vi "UMLEditor createWizardScriptFile.vi"(1 "localVariables":T3 {"ObjectHotspots"."HotSpot"."y" format="%.2f"; "ObjectHotspots"."HotSpot"."x" format="%.2f"; "NodesBounds"."height" format="%.2f"; "NodesBounds"."width" format="%.2f"; "NodesBounds"."y" format="%.2f"; "NodesBounds"."x" format="%.2f"; "offset"."y" format="%.2f"; "offset"."x" format="%.2f"; "gridSize" format="%.2f"; "dragStartBounds"."height" format="%.2f"; "dragStartBounds"."width" format="%.2f"; "dragStartBounds"."y" format="%.2f"; "dragStartBounds"."x" format="%.2f"; "dragStartPoint"."y" format="%.2f"; "dragStartPoint"."x" format="%.2f"; "rubberBandStart"."y" format="%.2f"; "rubberBandStart"."x" format="%.2f"; "lastMousePoint"."y" format="%.2f"; "lastMousePoint"."x" format="%.2f"; "zoom" format="%.2f"}, 2 "OnlySelectedNode(False)":bool, 5 "error in (no error)":errorcluster) -> (14 "localVariables":T3 {"ObjectHotspots"."HotSpot"."y" format="%.2f"; "ObjectHotspots"."HotSpot"."x" format="%.2f"; "NodesBounds"."height" format="%.2f"; "NodesBounds"."width" format="%.2f"; "NodesBounds"."y" format="%.2f"; "NodesBounds"."x" format="%.2f"; "offset"."y" format="%.2f"; "offset"."x" format="%.2f"; "gridSize" format="%.2f"; "dragStartBounds"."height" format="%.2f"; "dragStartBounds"."width" format="%.2f"; "dragStartBounds"."y" format="%.2f"; "dragStartBounds"."x" format="%.2f"; "dragStartPoint"."y" format="%.2f"; "dragStartPoint"."x" format="%.2f"; "rubberBandStart"."y" format="%.2f"; "rubberBandStart"."x" format="%.2f"; "lastMousePoint"."y" format="%.2f"; "lastMousePoint"."x" format="%.2f"; "zoom" format="%.2f"}, 15 "pathToScriptFile":path, 16 "Cancelled":bool, 17 "Class folder":path, 19 "error out":errorcluster)   [LabVIEW 2020]
doc: "Gets current diagram values"
uses:
  <resource>/Framework/Providers/Open_GDS/UML/UMLEditor/UMLEditor LocalVariablesType.ctl
  <resource>/Framework/Providers/Open_GDS/UML/AbstractNode_class/AbstractNode.lvclass
  <resource>/Framework/Providers/Open_GDS/UML/AbstractEdge_class/AbstractEdge.lvclass
  <resource>/Framework/Providers/Open_GDS/UML/Graphics_class/Graphics.lvclass
  <resource>/Framework/Providers/Open_GDS/UML/Grid_class/Grid.lvclass
  <resource>/Framework/Providers/Open_GDS/UML/UMLEditor/UMLEditor statesType.ctl
  <resource>/Framework/Providers/Open_GDS/UML/UMLEditor/UMLEditor tooltype.ctl
  <resource>/Framework/Providers/Open_GDS/UML/UMLEditor/UMLEditor_DiagramInfo.ctl
  <resource>/Framework/Providers/Open_GDS/UML/Graph_class/Graph.lvclass
  <resource>/Framework/Providers/Open_GDS/UML/General/Point/Point Point2D.ctl
  <resource>/Framework/Providers/Open_GDS/UML/General/Rectangle/Rectangle Rectangle2D.ctl
  <resource>/Framework/Providers/Open_GDS/UML/UMLEditor/UMLEditor ExportType.ctl
  <resource>/Framework/Providers/Open_GDS/UML/UMLEditor/UMLEditor FlattenCommandType.ctl
  <resource>/Framework/Providers/Open_GDS/UML/UMLEditor/UMLEditor ExecuteCommandType.ctl
  <resource>/Framework/Providers/Open_GDS/UML/ContextHelp/ContextHelp_EventType.ctl
  <resource>/Framework/Providers/Open_GDS/UML/UMLEditor/UMLEditor_HotSpotData.ctl
  <resource>/Framework/Providers/Open_GDS/UML/UMLEditor/UMLEditor_HotSpotType.ctl
  <resource>/Framework/Providers/Open_GDS/UML/UmlEditor_class/EventData.ctl
  <resource>/Framework/Providers/Open_GDS/UML/UMLEditor/UMLEditor GOOPWizardClassSpecification.ctl
  <resource>/Framework/Providers/Open_GDS/UML/ClassNode_class/ClassNode.lvclass
  C:/Program Files (x86)/National Instruments/LabVIEW 2020/resource/Framework/Providers/Open_GDS/UML/AbstractNode_class/AbstractNode.lvclass
  <resource>/Framework/Providers/Open_GDS/ClassProviders/Common/ScriptingFunctions/Scripting_ConnectorPanePatternType.ctl
  <resource>/Framework/Providers/Open_GDS/UML/ClassRelationshipEdge_class/ClassRelationshipEdge.lvclass
  <resource>/Framework/Providers/Open_GDS/ClassProviders/Provider_BaseClassInterface/ClassWriter_class/ClassWriter.lvclass
  <resource>/Framework/Providers/Open_GDS/UML/UMLEditor/UMLEditor_StoredPathes.ctl
  <resource>/Framework/Providers/Open_GDS/UML/InterfaceNode_class/InterfaceNode.lvclass
  <resource>/Framework/Providers/Open_GDS/UML/ContextHelp/ContextHelp_HelpTexts.ctl
  <resource>/Framework/Providers/Open_GDS/SubVIs/GOOP_ClassProviderClassType.ctl
  <resource>/Framework/Providers/Open_GDS/ClassProviders/Provider_BaseClassInterface/CreateClassData.ctl
  <resource>/Framework/Providers/Open_GDS/ClassProviders/Common/LvIcon_class/subvis/GDSLvIcon_TextDataType.ctl
  <resource>/Framework/Providers/Open_GDS/ClassProviders/Common/LvIcon_class/GDSLvIcon_WordCompressionType.ctl
  <resource>/Framework/Providers/Open_GDS/ClassProviders/Common/LvIcon_class/GDSLvIcon_TextAlignment.ctl
  <resource>/Framework/Providers/Open_GDS/ClassProviders/Common/LvIcon_class/GDSLvIcon_ClassColorTypes.ctl
  <resource>/Framework/Providers/Open_GDS/ClassProviders/Provider_BaseClassInterface/CreateInterfaceData.ctl
  <resource>/Framework/Providers/Open_GDS/ClassProviders/Provider_BaseClassInterface/ClassWriter_class/InterfaceMethodsToCreate.ctl
  <resource>/Framework/Providers/Open_GDS/ClassProviders/Common/CommonVIs/CommonVIs_AttributeType.ctl
  <resource>/Framework/Providers/Open_GDS/ClassProviders/Common/CommonVIs/CommonVIs_AttributeDataType.ctl
  <resource>/Framework/Providers/Open_GDS/ClassProviders/Common/String/GDSString_AccessScopeModifierType.ctl
  <resource>/Framework/Providers/Open_GDS/UML/ClassNode_class/ExternalSetTypes.ctl
  <resource>/Framework/Providers/Open_GDS/ClassProviders/Common/CommonVIs/CommonVIs_ClassNamePathType.ctl
  <resource>/Framework/Providers/Open_GDS/UML/ReversedEngineering/private/ReversedEngineering SyncUmlFromCodeActions.ctl
  <resource>/Framework/Providers/Open_GDS/ClassProviders/Common/ScriptingFunctions/Scripting.lvclass
  <resource>/Framework/Providers/Open_GDS/ClassProviders/Common/InterfaceLibrary/InterfaceLibrary.lvlib
  <resource>/Framework/Providers/Open_GDS/UML/UmlEditor_class/UmlEditor.lvclass
panel:
  out "Tab":enum32{"Create", "Config"}(tab)
  in  "InterfaceFolderSuffix":string="_class" caption="Interface folder suffix"
  in  "ModifyProviders":bool
  in  "Connector Pane Pattern":T1=2 items=["4x4x4", "5x6x5", "6x8x6"]
  in  "_UseLLB":bool
  in  "_CurrentClassProvider":u16(ring) caption="Class provider to use:" items=["By Reference DVR (GOOP4)", "LVClass by value", "By Reference (GOOP3)"]
  in  "Project":u16(ring) caption="Select project to add classes to" items=["Interface2.lvproj"]
  in  "Help":bool
  in  "ClassFolderSuffix":string="_class" caption="Class folder suffix"
  in  "Cancel 2":bool
  in  "CreateClasses":bool
  in  "down":bool
  in  "up":bool
  in  "ClassPath":path caption="Path for created classes (ignored for classes with a defined class path)"
  in  "Classes":T2(array[cluster])
  out "Class creation progress":i32(listbox)
  in  "Use":bool=TRUE
  out "classes":T15[](array[typedef]) {"ClassType" items=["Standard class", "Sub class from an existing base class", "Clone class from an existing class"]; "Methods"."Method Type" items=["Reading", "Modifying", "Class method - Non Modifying", "Class method - Reading", "Class method - Modifying", "Constructor", "Destructor", "Type Def"]}
  in  "ScriptfilePath":path caption="Path to store Scriptfile"
  # "LLBs"
  # "Directories"
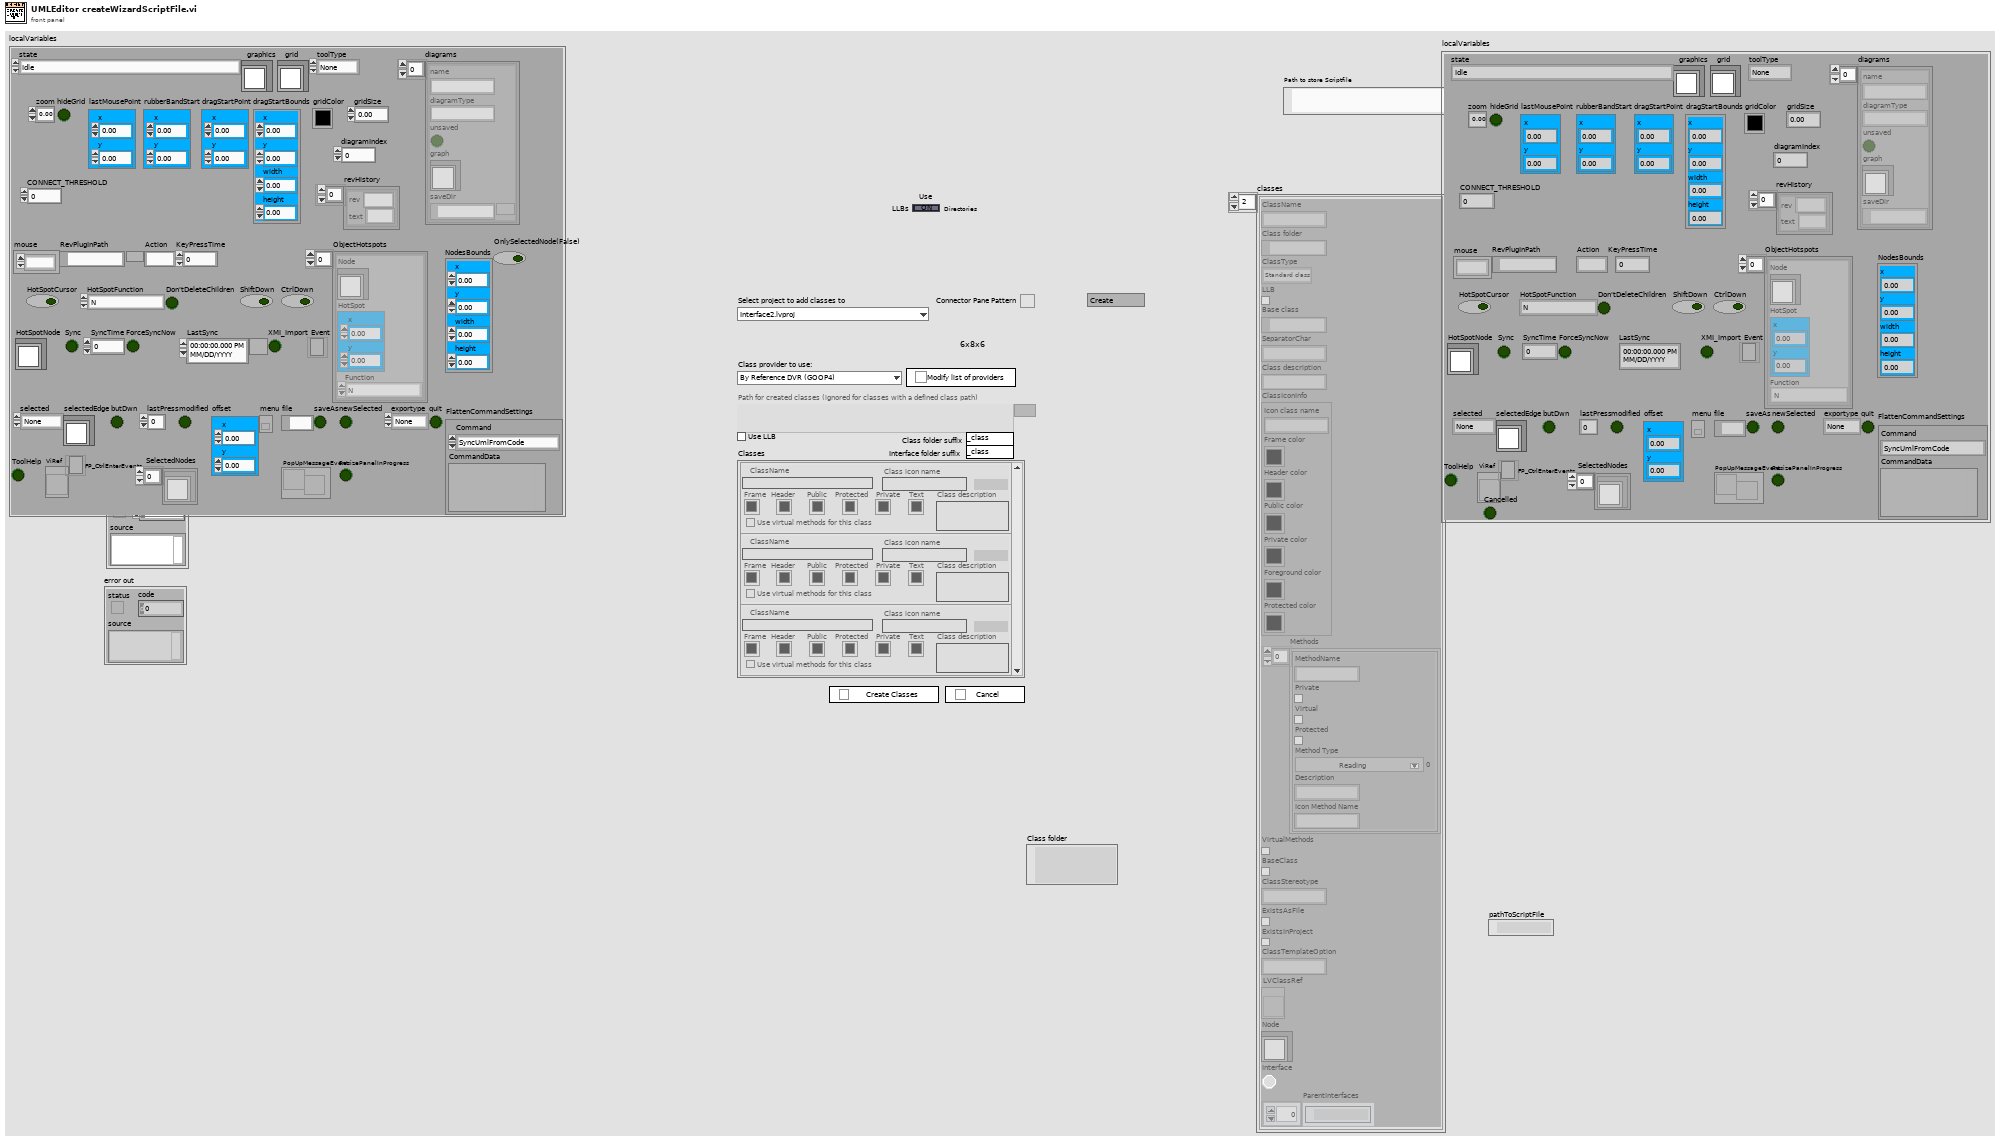
[diagram p1: front panel]
types:
  T1 = typedef "Scripting_ConnectorPanePatternType.ctl" = u16
  T2 = cluster{"ClassName":string, "Class icon name":string, "Frame":u32, "Header":u32, "Public":u32, "Protected":u32, "Private":u32, "Text":u32, "text":string, "Class description":string, "UseVirtuals":bool, "ClassIdex":i32}[]
  T3 = typedef "UMLEditor LocalVariablesType.ctl" = cluster{"state":T4, "graphics":refnum<class "Graphics.lvclass">, "grid":refnum<class "Grid.lvclass">, "toolType":T5, "diagramIndex":i32, "diagrams":T6[], "zoom":dbl, "hideGrid":bool, "lastMousePoint":T7, "rubberBandStart":T7, "dragStartPoint":T7, "dragStartBounds":T8, "gridColor":u32, "gridSize":dbl, "CONNECT_THRESHOLD":i32, "selected":T5, "selectedEdge":refnum<class "AbstractEdge.lvclass">, "butDwn":bool, "lastPress":u32, "modified":bool, "offset":T7, "menu":refnum<k9>, "file":path, "saveAs":bool, "newSelected":bool, "exportype":T9, "quit":bool, "revHistory":cluster{"rev":string, "text":string}[], "FlattenCommandSettings":T10, "PopUpMessageEvent":T12, "ResizePanelInProgress":bool, "NodesBounds":T8, "ToolHelp":bool, "ViRef":refnum<vi>, "FP_CtrlEnterEvents":refnum<event-registration>, "SelectedNodes":refnum<class "AbstractNode.lvclass">[], "mouse":refnum<k1>, "RevPlugInPath":path, "Action":string, "KeyPressTime":u32, "ObjectHotspots":T13[], "HotSpotCursor":bool, "HotSpotFunction":T14, "Don'tDeleteChildren":bool, "ShiftDown":bool, "CtrlDown":bool, "HotSpotNode":refnum<class "AbstractNode.lvclass">, "Sync":bool, "SyncTime":u32, "ForceSyncNow":bool, "LastSync":timestamp, "XMI_Import":bool, "Event":refnum<event-registration>}
  T4 = typedef "UMLEditor statesType.ctl" = enum16{"Idle", "CheckLicense", "revHistory", "Init", "Init2", "EditSelected", "RemoveSelected", "PaintComponent", "ChangeZoom", "ChangeGridSize", "Open", "Close", "Save", "ExportPicture", "Export", "Repaint", "Error", "Exit", "QUIT", "CreateScript", "ExecuteScript", "ClassReversedEngineering", "PlugInReverseEngineering", "StateReversedEngineering", "AutoPlace", "ExecuteCommand", "OpenClass", "SyncAll", "StraightenAssociation", "Copy", "Paste", "AddNodeFromProjectTree", "AddNodeFromProjectTree+SyncAll", "PanAndRepaint", "Init3", "CopyPaste", "ApplyDesignPattern", "AnalyseViInStateDiagram", "AutoSync"}
  T5 = typedef "UMLEditor tooltype.ctl" = enum16{"None", "Node", "Edge"}
  T6 = typedef "UMLEditor_DiagramInfo.ctl" = cluster{"name":string, "diagramType":string, "unsaved":bool, "graph":refnum<class "Graph.lvclass">, "saveDir":path}
  T7 = typedef "Point Point2D.ctl" = cluster{"x":dbl, "y":dbl}
  T8 = typedef "Rectangle Rectangle2D.ctl" = cluster{"x":dbl, "y":dbl, "width":dbl, "height":dbl}
  T9 = typedef "UMLEditor ExportType.ctl" = enum16{"None", "Printer", "png", "jpg", "roseUML"}
  T10 = typedef "UMLEditor FlattenCommandType.ctl" = cluster{"Command":T11, "CommandData":variant}
  T11 = typedef "UMLEditor ExecuteCommandType.ctl" = enum16{"SyncUmlFromCode", "SyncCodeFromUML", "OpenClass", "OpenFile", "CreateClass", "CreateVI", "OpenClassAttribute", "LocateInProject", "GraphExecute"}
  T12 = typedef "ContextHelp_EventType.ctl" = refnum<user-event>
  T13 = typedef "UMLEditor_HotSpotData.ctl" = cluster{"Node":refnum<class "AbstractNode.lvclass">, "HotSpot":T7, "Function":T14}
  T14 = typedef "UMLEditor_HotSpotType.ctl" = enum16{"N", "NE", "E", "SE", "S", "SW", "W", "NW", "Expand", "Collaps"}
  T15 = typedef "UMLEditor GOOPWizardClassSpecification.ctl" = cluster{"ClassName":string, "Class folder":path, "ClassType":i32, "LLB":bool, "Base class":path, "SeparatorChar":string, "Class description":string, "ClassIconInfo":cluster{"Icon class name":string, "Frame color":u32, "Header color":u32, "Public color":u32, "Private color":u32, "Foreground color":u32, "Protected color":u32}, "Methods":cluster{"MethodName":string, "Private":bool, "Virtual":bool, "Protected":bool, "Method Type":i32, "Description":string, "Icon Method Name":string}[], "VirtualMethods":bool, "BaseClass":bool, "ClassStereotype":string, "ExistsAsFile":bool, "ExistsInProject":bool, "ClassTemplateOption":string, "LVClassRef":refnum<vi>, "Node":refnum<class "ClassNode.lvclass">, "Interface":bool, "ParentInterfaces":path[]}
  T16 = cluster{"graph":refnum<class "Graph.lvclass">, "nodes":refnum<class "ClassNode.lvclass">[], "InheritEdges":refnum<class "ClassRelationshipEdge.lvclass">[], "classes":T15[], "subNodes":refnum<class "ClassNode.lvclass">[], "classGeneratorPath":path, "scriptFilePath":path, "AllNodes":refnum<class "ClassNode.lvclass">[], "CompAggEdges":refnum<class "ClassRelationshipEdge.lvclass">[], "baseNodes":refnum<class "ClassNode.lvclass">[], "Types":refnum<class "ClassNode.lvclass">[], "cancel":bool, "ClassProvider":i32, "My Computer":refnum<vi>, "ClassWriterRef":refnum<class "ClassWriter.lvclass">, "G4":bool, "Providers":string[], "InterfaceEdges":refnum<class "ClassRelationshipEdge.lvclass">[]}
  T17 = typedef "UMLEditor_StoredPathes.ctl" = enum16{"LastSearchPath", "QueuedArrayStateVI", "ClassBasePath", "ViTemplatePath", "ApplicationTemplatePath", "IniFilePath", "WizDir", "RevPlugInPath"}
  T18 = typedef "ContextHelp_HelpTexts.ctl" = enum16{"None(Hide)", "Default", "Help", "Welcome", "GettingStarted", "ClassDiagram_Help", "SequenceDiagram_Help", "UseCaseDiagram_Help", "BSelect", "BClass", "BInterface", "BPackage", "BNote", "BDependency", "BInheritance", "BInterfaceImplementation", "BAssociation", "BAggregation", "BCompAggregation", "BNoteConnector", "BObject", "BActionBar", "BCall", "BSystem", "BActor", "BUseCase", "BGeneralization", "BIncludes", "BExtends", "BUseCaseDiagramAssociation", "ClassRelationshipEdge editDialog_Bent Style", "ClassRelationshipEdge editDialog_RelationType", "ClassRelationshipEdge editDialog_Reverse association", "ClassRelationshipEdge editDialog_Start label", "ClassRelationshipEdge editDialog_Middle label", "ClassRelationshipEdge editDialog_End label", "UMLEditor reversedEngineering_Pathes", "ReversedEngineering StateReverseDialog_Help", "ReversedEngineering StateQueuedSettings_Help", "UMLEditor reversedEngineering_AddTopVIs", "UMLEditor reversedEngineering_AddClasses", "UMLEditor reversedEngineering_AddDirs", "UMLEditor reversedEngineering_Recursively", "UMLEditor reversedEngineering_Remove", "UMLEditor reversedEngineering_ClearList", "UMLEditor reversedEngineering_HideSubAss", "UMLEditor reversedEngineering_CreateTypes", "UMLEditor reversedEngineering_OnlyInheritance", "UMLEditor reversedEngineering_CreateApplication", "UMLEditor reversedEngineering_OK", "UMLEditor reversedEngineering_Cancel", "UMLEditor reversedEngineering_Help", "UMLEditor createWizardScriptFile_ScriptfilePath", "UMLEditor createWizardScriptFile_ClassPath", "UMLEditor createWizardScriptFile_Use", "UMLEditor createWizardScriptFile_PrivateDirName", "UMLEditor createWizardScriptFile_DirAppend", "UMLEditor createWizardScriptFile_Separator Character", "UMLEditor createWizardScriptFile_OK", "UMLEditor createWizardScriptFile_Cancel", "UMLEditor createWizardScriptFile_Help", "ClassNode editDialog_Class Name", "InterfaceNode editDialog_Class Name", "ClassNode editDialog_Attribute", "ClassNode editDialog_Methods", "InterfaceNode editDialog_Methods", "ClassNode editDialog_connection", "InterfaceNode editDialog_connection", "ClassNode editDialog_StereoType", "ClassNode editDialog_ShowAttrib", "ClassNode editDialog_ShowMethods", "ClassNode editDialog_ClassPath", "ClassNode editDialog_AddAttribute", "ClassNode editDialog_AddMethod", "InterfaceNode editDialog_AddMethod", "ClassNode AttributeGuide_AttributeName", "ClassNode AttributeGuide_Array?", "ClassNode AttributeGuide_Data Type", "ClassNode AttributeGuide_RefName", "ClassNode AttributeGuide_Preview", "ClassNode AttributeGuide_OK", "ClassNode AttributeGuide_Cancel", "ClassNode MethodGuide_Visibility", "ClassNode MethodGuide_Method Name", "ClassNode MethodGuide_Preview", "ClassNode MethodGuide_OK", "ClassNode MethodGuide_Cancel", "CallNode EditCallProperties_AllButtons", "ObjectNode EditObjectlProperties_AllButtons", "ActorNode EditActorProperties_AllButtons", "UseCaseRelationshipNode EditUseCaselProperties_AllButtons", "UseCaseNode EditUseCaselProperties_AllButtons", "SystemNode EditSystemProperties_AllButtons", "ReversedEngineering UpdateAttributes_AllButtons", "StateNode editDialog_AllButtons", "StateTransition editDialog_AllButtons", "ArrangeNodes Main_Picture", "ArrangeNodes Main_Zoom", "ArrangeNodes Main_Auto Zoom", "ArrangeNodes Main_shorten", "ArrangeNodes Main_Min Length", "ArrangeNodes Main_Max Length", "ArrangeNodes Main_increase", "ArrangeNodes Main_decrease", "ArrangeNodes Main_Shake", "ArrangeNodes Main", "BState", "BInitialState", "BFinalState", "BStateTransition", "StateDiagram_Help", "StateDiagram_PropertiesAllButtons", "ReversedEngineering StateReverseDialog_ClearStates", "ReversedEngineering StateReverseDialog_UseQueuedStateMachines", "ReversedEngineering StateReverseDialog_QueuedSettings", "ReversedEngineering StateReverseDialog_SearchForVIs", "ReversedEngineering StateReverseDialog_SearchCriteria", "OptionsDialog_ClassBasePath", "OptionsDialog_VIPath", "OptionsDialog_ApplicationPath", "OptionsDialog_WizDir", "OptionsDialog_IniFilePath", "OptionsDialog_DefineColors", "OptionsDialog_Help", "OptionsDialog_CreateTypes", "ClassRelationshipEdge editDialog_SplitWire"}
  T19 = typedef "GOOP_ClassProviderClassType.ctl" = enum16{"ClassWriter", "ClassReader"}
  T20 = typedef "GDSLvIcon_ClassColorTypes.ctl" = cluster{"Frame":u32, "Header Text Color":u32, "Header Background":u32, "BodyBackgroundPublic":u32, "BodyBackgroundProtected":u32, "BodyBackgroundPrivate":u32, "Body Text Color":u32, "Frame thickness":u8, "ProtectedPrivateSame":bool, "Icon Header Size":u8, "Font Compression":enum16{"Auto", "On", "Off"}, "CapitalOnly":bool}
  T21 = typedef "GDSLvIcon_TextDataType.ctl" = cluster{"Text":string, "Allow Only Capital Chars":bool, "Compression":T22, "Alignment":T23}
  T22 = typedef "GDSLvIcon_WordCompressionType.ctl" = enum16{"Auto", "On", "Off"}
  T23 = typedef "GDSLvIcon_TextAlignment.ctl" = enum16{"Center", "Left", "Right"}
  T24 = typedef "ClassWriter.lvclass/CreateClassData.ctl" = cluster{"ClassName":string, "ClassFolder":path, "ClassDescription":string, "ClassTemplateOptions":string, "BaseClass(ProjectStringPath or LvClassFilePath)":variant, "ExtraCreateParameters":variant, "FolderSuffix":string, "ParentInterfaces":path[]}
  T25 = typedef "ClassWriter.lvclass/CreateInterfaceData.ctl" = cluster{"InterfaceName":string, "InterfaceFolder":path, "InterfaceDescription":string, "FolderSuffix":string, "MethodsToCreate":T26[], "ParentInterfaces":path[]}
  T26 = typedef "ClassWriter.lvclass/InterfaceMethodsToCreate.ctl" = cluster{"Name":string, "Description":string, "MethodsArgumentsIn":T27[], "MethodsArgumentsOut":T27[], "DecendantsMustOverride":bool}
  T27 = typedef "CommonVIs_AttributeType.ctl" = cluster{"Name":string, "DataType":T28, "ArrayDim":i32, "CtrlPath":path, "DataTypeString":string, "AccessScope":T29, "InitialData":variant}
  T28 = typedef "CommonVIs_AttributeDataType.ctl" = enum16{"UINT8", "INT8", "UINT16", "INT16", "UINT32", "INT32", "UINT64", "INT64", "SGL", "DBL", "EXT", "CSG", "CDB", "CXT", "TimeStamp", "STRING", "PATH", "BOOL", "ENUM", "RefNum", "VIRefNum", "LabVIEW Class", "Cluster", "Variant", "TypeDef", "Waveform", "LabVIEW Object", "Other", "void", "Set", "Map"}
  T29 = typedef "GDSString_AccessScopeModifierType.ctl" = enum16{"public", "private", "protected", "internal"}
  T30 = typedef "ClassNode.lvclass/ExternalSetTypes.ctl" = enum16{"Name", "Attributes", "Methods", "Position", "ShowMethods", "ShowAttributes", "ClassPath"}
  T31 = typedef "CommonVIs_ClassNamePathType.ctl" = cluster{"ClassNamn":string, "ClassPath":path, "InterfaceClass":bool}
  T32 = typedef "ReversedEngineering SyncUmlFromCodeActions.ctl" = enum16{"GetAttributes&MethodsFromCode", "GetAll"}
  T33 = typedef "UMLEditor_DiagramType.ctl" = string
  T34 = typedef "BaseProvider_IniFileSettings.ctl" = cluster{"ClassFolderSuffix":string, "InterfaceFolderSuffix":string, "InterfaceIcon":string, "FileNamingOption":T35}
  T35 = typedef "BaseProvider_FileNamingOption.ctl" = enum16{"CamelCase", "Space", "Underscore"}
  T36 = typedef "CommonVIs_StereoType.ctl" = enum16{"None", "TYPE", "ENUM", "ABSTRACT", "ACTOR", "GUI", "SINGLETON", "SIGNAL", "BOUNDARY", "ENTITY", "CONTROL", "LEGACY", "APPLICATION", "VI", "LVLIB", "INTERFACE"}
  T37 = cluster{"MethodName":string, "Private":bool, "Virtual":bool, "Protected":bool, "Method Type":i32, "Description":string, "Icon Method Name":string}[]
  T38 = cluster{"MethodName":string, "Private":bool, "Virtual":bool, "Protected":bool, "Method Type":i32, "Description":string, "Icon Method Name":string}
  T39 = cluster{"ClassName":string, "Class icon name":string, "Frame":u32, "Header":u32, "Public":u32, "Protected":u32, "Private":u32, "Text":u32, "text":string, "Class description":string, "UseVirtuals":bool, "ClassIdex":i32}
  T40 = enum16{"Left Button", "Center Button", "Right Button", "Window Close"}
  T41 = enum32{"existing file", "new file", "new or existing file", "existing dir", "new dir", "new or existing dir", "existing file (use LLBs)", "new file (use LLBs)", "new or existing file (use LLBs)", "new or existing file or directory (use LLBs)"}
  T42 = typedef "ContextHelp_ShowType.ctl" = cluster{"Header":string, "Picture":picture, "Text":string}
  T43 = typedef "GOOP_WireConfigurationType.ctl" = cluster{"Edge thickness":i32, "Edge color":u32, "Center thickness":i32, "Center pattern":T44, "CenterColor1":u32, "CenterColor2":u32, "Tunnels and terminals colors":u32}
  T44 = typedef "GOOP_WirePattern.ctl" = enum16{"Solid", "Large dash", "Small dash"}
  T45 = typedef "ClassWriter.lvclass/ClassTemplateType.ctl" = cluster{"TemplateIdName":string, "TemplateUserDialogName":string, "OnlySubClassTemplate":bool, "CanDeriveFromTheseTemplateIDs":string[], "ClassSuffix":string, "Description":string, "LvLibTemplate":bool}
  T46 = cluster{"Icon class name":string, "Frame color":u32, "Header color":u32, "Public color":u32, "Private color":u32, "Foreground color":u32, "Protected color":u32}
  T47 = enum32{"invalid VI type", "Standard VI", "Control VI", "Global VI", "Polymorphic VI", "Configuration VI", "SubSystem", "Facade VI", "Method VI", "Statechart Diagram VI"}
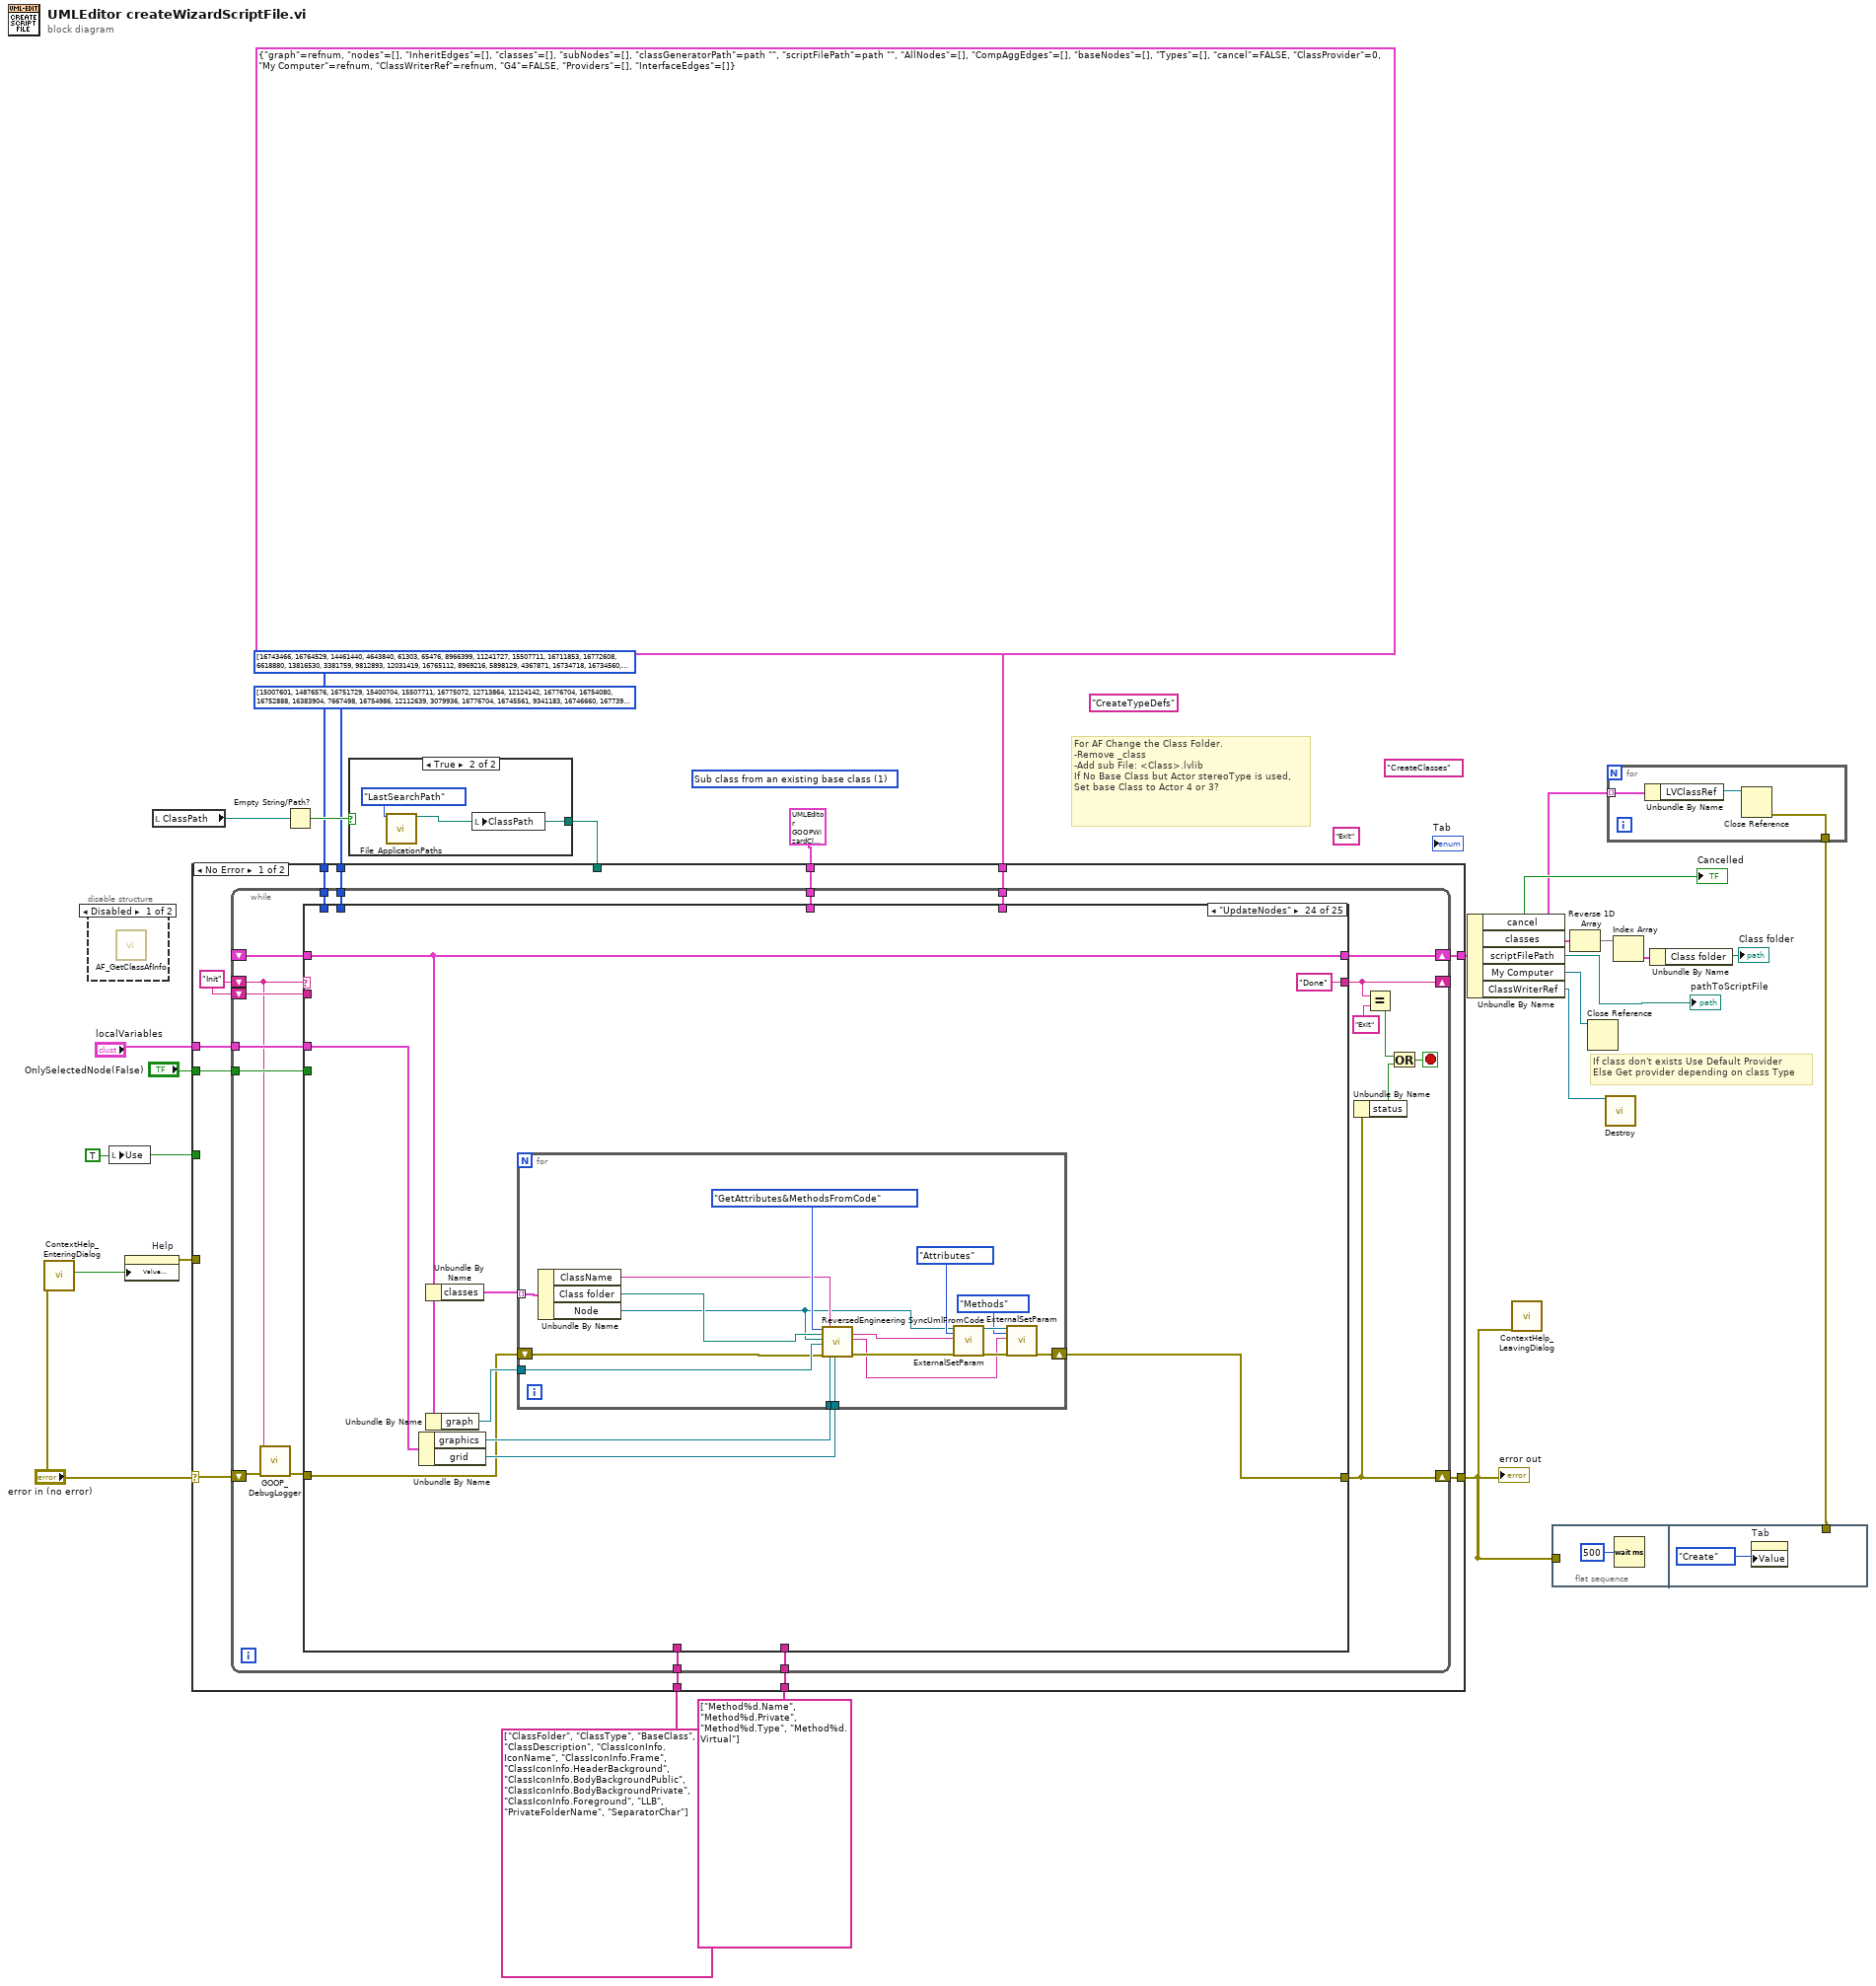
[diagram p0: block diagram]
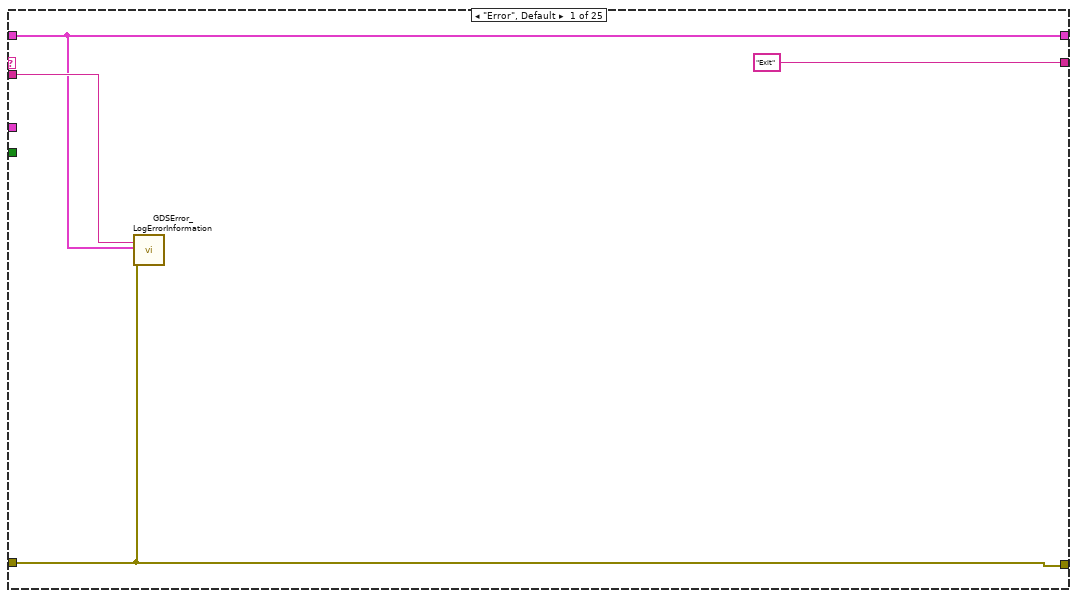
[diagram p4: hidden frame]
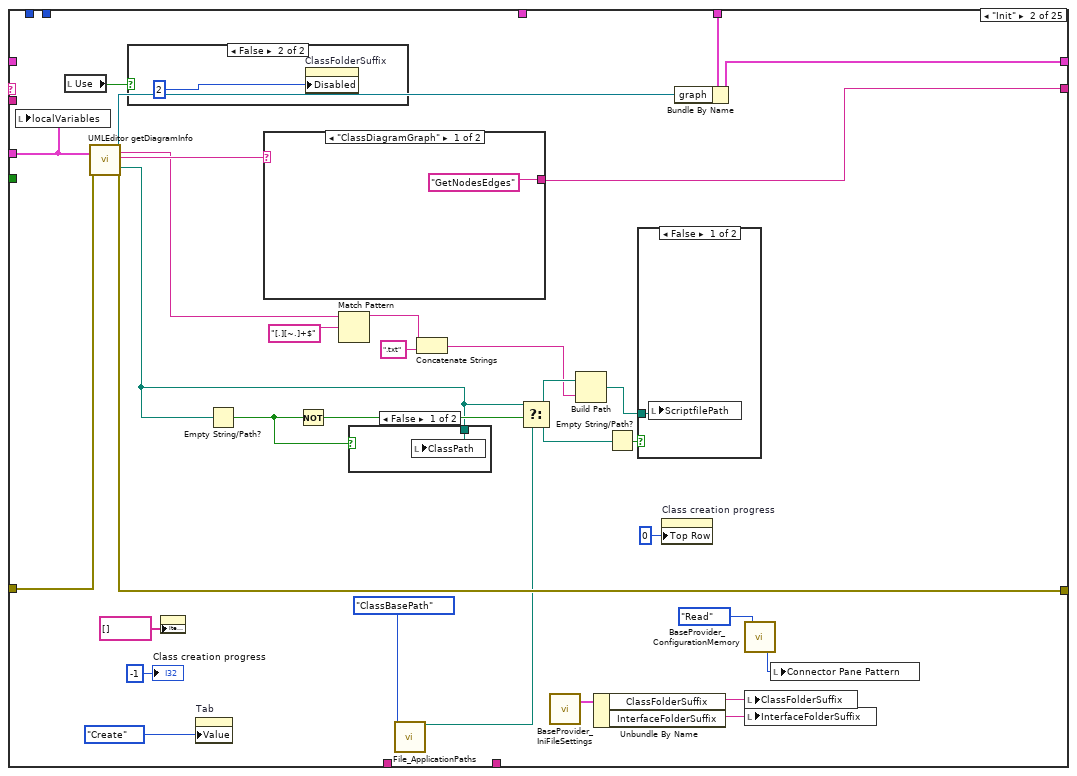
[diagram p5: hidden frame]
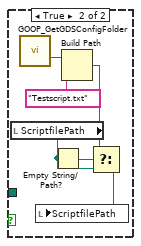
[diagram p6: hidden frame]
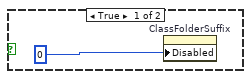
[diagram p8: hidden frame]
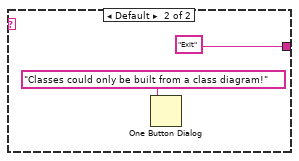
[diagram p9: hidden frame]
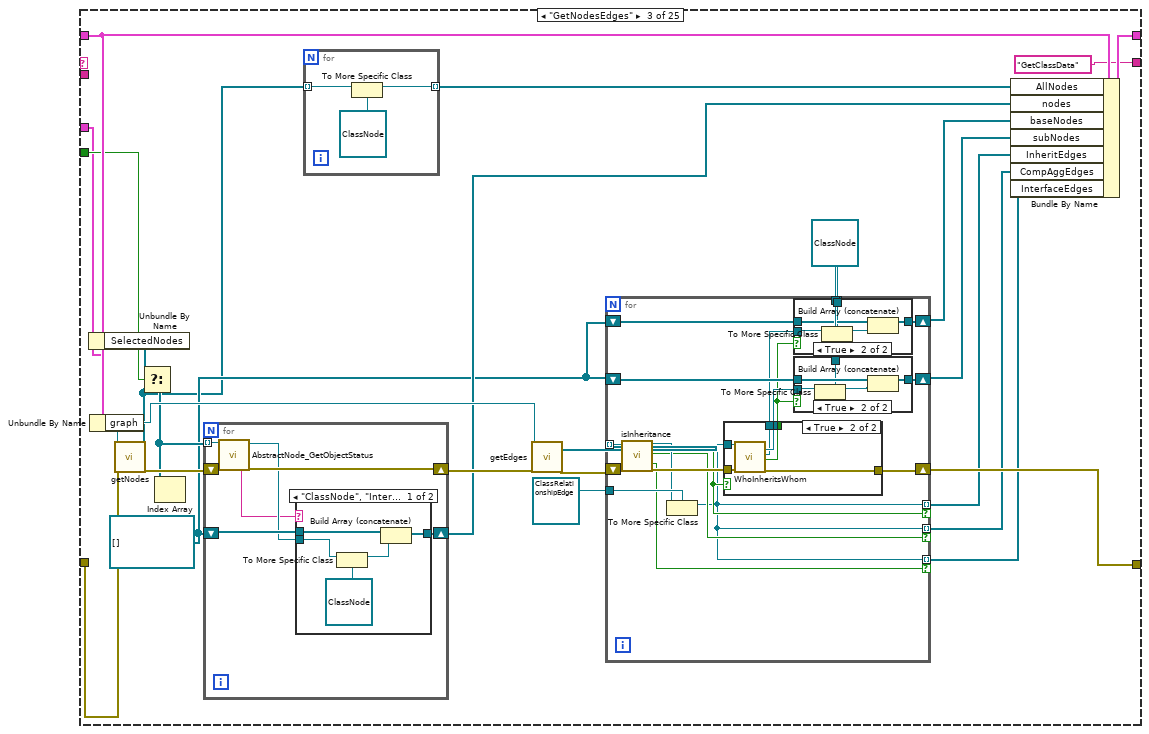
[diagram p10: hidden frame]
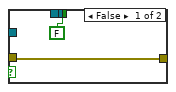
[diagram p13: hidden frame]
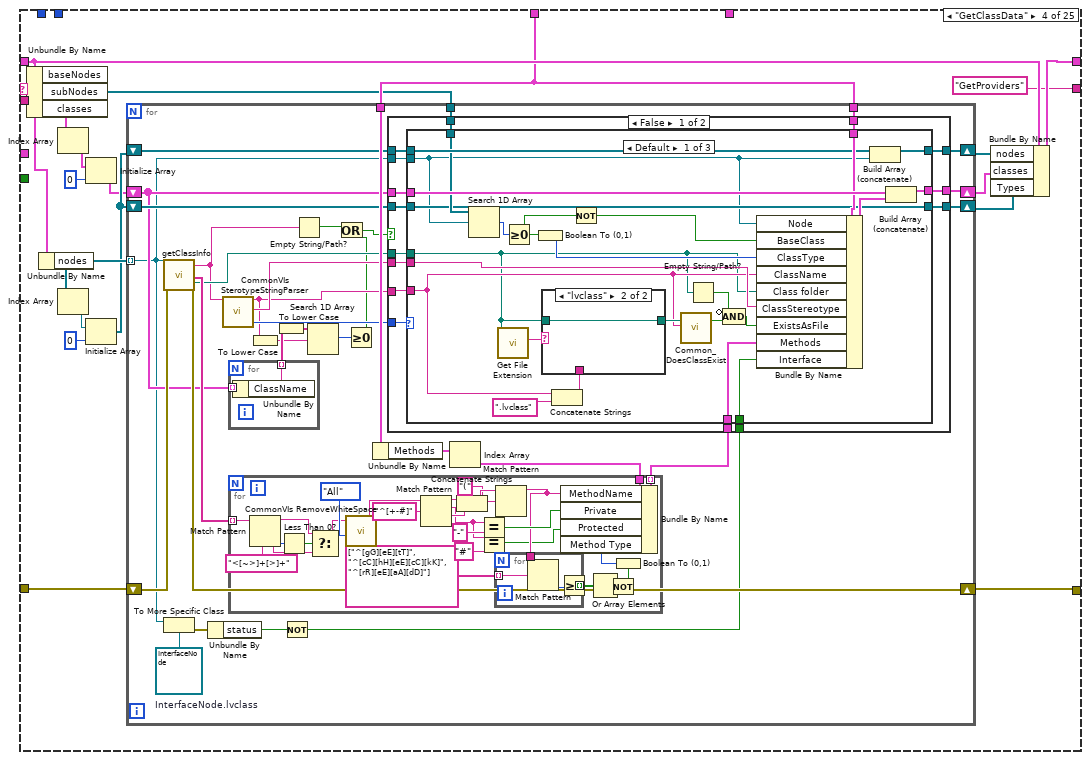
[diagram p15: hidden frame]
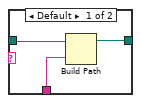
[diagram p16: hidden frame]
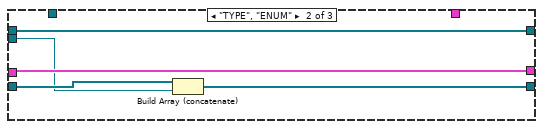
[diagram p17: hidden frame]
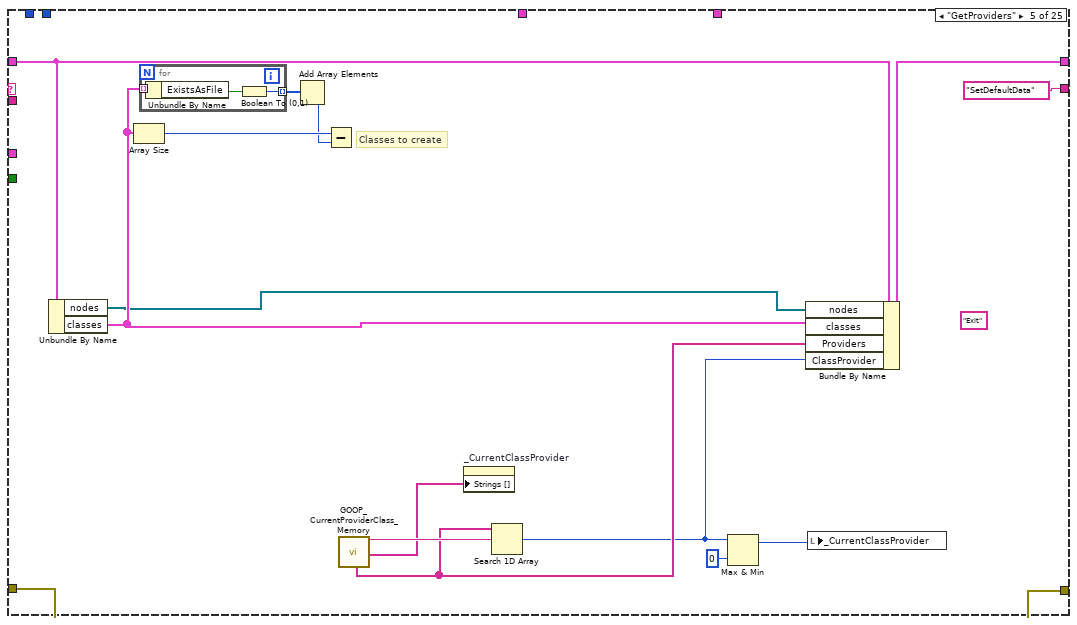
[diagram p20: hidden frame]
diagram:
  (unwired) 1 items=["Standard class", "Sub class from an existing base class", "Clone class from an existing class"] ("ClassType")
  (unwired) "CreateClasses"
  (unwired) "Exit" ("y")
  (unwired) "CreateTypeDefs" ("y")
  w8 = TRUE ("Use")
  # "For AF Change the Class Folder.\n-Remove _class\n-Add sub File: <Class>.lvlib\nIf No Base Class but Actor stereoType is used,\nSet base Class to Actor 4 or 3?"
  # "If class don't exists Use Default Provider\nElse Get provider depending on class Type"
  n1 = call <resource>:"ContextHelp_EnteringDialog.vi"("error in (no error)"="error in (no error)") -> ("HelpStatus"=w16:bool)  [unwired: 2 in, 16 out]
  n2 = disable-structure shown="Disabled" {
    frame Disabled {
      n3 = call <resource>:"AF_GetClassAfInfo.vi"() -> ()  [unwired: 6 in, 6 out]
    }
    frame Enabled {
    }
  }
  n4 = local write "Use"(w8) -> ()
  n5 = property on="Help" class="Bool (strict)"("Value (Signaling)"=w16) -> (error out=w1:errorcluster)  [unwired: 2 in, 1 out]
  n6 = local read "ClassPath"() -> (w13:path)
  n7 = Empty String/Path?(string/path=w13) -> (empty?=w12:bool)
  n8 = case shown="True" w12 {
    tunnel: [_ w27] -> w11
    frame False {
    }
    frame True {
      n9 = call <resource>:"File_ApplicationPaths.vi"("PathName"=UMLEditor_StoredPathes."LastSearchPath" ("UMLPathes")) -> ("Path Out"=w27:path)  [unwired: 3 in, 15 out]
      n10 = local write "ClassPath"(w27) -> ()
    }
  }
  n11 = case shown="No Error" "error in (no error)" {
    selector: "error in (no error)" -> [w38 w1735]
    tunnel: [w39 w1735] -> w4
    tunnel: "localVariables" -> [w40 _]
    tunnel: T15 {"ClassName"="", "Class folder"=path "", "ClassType"=0, "LLB"=FALSE, "Base class"=path "", "SeparatorChar"="", "Class description"="", "ClassIconInfo"={"Icon class name"="", "Frame color"=0, "Header color"=0, "Public color"=0, "Private color"=0, "Foreground color"=0, "Protected color"=0}, "Methods"=[], "VirtualMethods"=FALSE, "BaseClass"=FALSE, "ClassStereotype"="", "ExistsAsFile"=FALSE, "ExistsInProject"=FALSE, "ClassTemplateOption"="", "LVClassRef"=refnum, "Node"=refnum, "Interface"=FALSE, "ParentInterfaces"=[]} ("Class Info") -> [w37 _]
    tunnel: string[] ["Method%d.Name", "Method%d.Private", "Method%d.Type", "Method%d.Virtual"] -> [w36 _]
    tunnel: string[] ["ClassFolder", "ClassType", "BaseClass", "ClassDescription", "ClassIconInfo.IconName", "ClassIconInfo.Frame", "ClassIconInfo.HeaderBackground", "ClassIconInfo.BodyBackgroundPublic", "ClassIconInfo.BodyBackgroundPrivate", "ClassIconInfo.Foreground", "LLB", "PrivateFolderName", "SeparatorChar"] -> [w35 _]
    tunnel: [w34 _] -> w22
    tunnel: "OnlySelectedNode(False)" -> [w33 _]
    tunnel: w11 -> [_ _]
    tunnel: u32[] [16743466, 16764529, 14461440, 4643840, 61303, 65476, 8966399, 11241727, 15507711, 16711853, 16772608, 6618880, 13816530, 3381759, 9812893, 12031419, 16765112, 8969216, 5898129, 4367871, 16734718, 16734560, 5856767, 13140224, 16759480] -> [w32 _]
    tunnel: u32[] [15007601, 14876576, 16751729, 15400704, 15507711, 16775072, 12713864, 12124142, 16776704, 16754080, 16752888, 16383904, 7667498, 16754986, 12112639, 3079936, 16776704, 16745561, 9341183, 16746660, 16773906, 2792191, 16762993, 5766954, 16318226] -> [w31 _]
    tunnel: w8 -> [_ _]
    tunnel: T16 {"graph"=refnum, "nodes"=[], "InheritEdges"=[], "classes"=[], "subNodes"=[], "classGeneratorPath"=path "", "scriptFilePath"=path "", "AllNodes"=[], "CompAggEdges"=[], "baseNodes"=[], "Types"=[], "cancel"=FALSE, "ClassProvider"=0, "My Computer"=refnum, "ClassWriterRef"=refnum, "G4"=FALSE, "Providers"=[], "InterfaceEdges"=[]} ("local") -> [w29 _]
    tunnel: w1 -> [_ _]
    frame No Error {
      w30 = "Init"
      n12 = while {
        shift-right: [w57] -> w39
        shift-left: w38 -> [w44]
        shift-right: [w55] -> _
        shift-left: w30 -> [w42]
        tunnel: w40 -> [w60]
        shift-right: [w59] -> w34
        shift-left: _ -> [w58]
        tunnel: w37 -> [w51]
        tunnel: w36 -> [w50]
        tunnel: w35 -> [w49]
        tunnel: w33 -> [w48]
        tunnel: w32 -> [w47]
        tunnel: w31 -> [w46]
        shift-left: w30 -> [w45]
        tunnel: w29 -> [w41]
        stop <- w52 stop-if-true
        n13 = call <resource>:"GOOP_DebugLogger.vi"("error in (no error)"=w44, "State"=w42) -> ("error out"=w43:errorcluster)  [unwired: 7 in, 2 out]
        n14 = case shown="\"UpdateNodes\"" w42 {
          selector: w42 -> [_ _ _ _ _ _ _ _ _ _ _ _ _ _ _ _ _ _ w1249 _ _ w1610 _ _ _]
          tunnel: w43 -> [w61 w95 w129 w200 w336 w350 w407 w424 w470 w649 w672 w751 w913 w954 w1011 w1074 w1144 w1203 w1258 w1484 w1530 w1617 w1675 w1707 w1732]
          tunnel: [w61 w90 w128 w198 w336 w350 w407 w422 w470 w629 w672 w750 w905 w953 w1010 w1073 w1144 w1203 w1253 w1475 w1532 w1618 w1674 w1706 w1732] -> w57
          tunnel: w60 -> [_ w81 w119 _ _ _ _ _ _ _ _ _ _ _ _ _ _ _ _ w1477 _ _ _ w1705 _]
          tunnel: [w62 w92 w127 w201 w340 w361 w404 w417 w467 w644 w678 w753 w899 w956 w1012 w1075 w1142 w1201 w1252 w1472 w1538 w1615 w1677 w1708 w1733] -> w59
          tunnel: ["Exit" w93 "GetClassData" "GetProviders" "SetDefaultData" "ClassPathVisible" "CheckProject" w425 w465 "UpdatePath&Color" "UpdateBaseClasses" w742 "CheckForClassTemplateToUse(Stereotype)" ("y") "UpdateAfStereoTypeWithNoBaseClass" "UpdateAfClassTemplate" "GetParentInterfaces" "ArrangeCreationOrder" "CreateClasses" "UpdateClassPathInDiagramClasses" ("y") w1478 w1537 "FixMethods" ("y") "UpdateNodes" ("y") "Done" ("y") "Exit" ("y")] -> w55
          tunnel: w58 -> [w62 _ w126 w202 w339 w363 w405 w417 w466 w650 w677 w754 w901 w957 w1013 w1076 w1136 w1197 w1250 w1473 w1538 w1615 w1677 w1708 w1733]
          tunnel: w51 -> [_ _ _ w199 _ _ _ _ _ _ _ _ _ _ _ _ _ _ _ _ _ _ _ _ _]
          tunnel: w50 -> [_ _ _ _ _ _ _ _ _ _ _ _ _ _ _ _ _ _ _ _ _ _ _ _ _]
          tunnel: w49 -> [_ _ _ _ _ _ _ _ _ _ _ _ _ _ _ _ _ _ _ _ _ _ _ _ _]
          tunnel: w48 -> [_ _ w121 _ _ _ _ _ _ _ _ w745 _ _ _ _ _ _ _ _ _ _ _ _ _]
          tunnel: w47 -> [_ _ _ _ _ w354 _ _ _ _ _ _ _ _ _ _ _ _ _ _ _ _ _ _ _]
          tunnel: w46 -> [_ _ _ _ _ w353 _ _ _ _ _ _ _ _ _ _ _ _ _ _ _ _ _ _ _]
          tunnel: w45 -> [w63 _ _ _ _ _ _ _ _ _ _ _ _ _ _ _ _ _ _ _ w1531 _ _ _ _]
          tunnel: w41 -> [_ w70 _ _ _ _ _ _ _ _ _ _ _ _ _ _ _ _ _ _ _ _ _ _ _]
          frame "Error", Default {
            n15 = call <resource>:"GDSError_LogErrorInformation.vi"("State"=w63, "LocalVariableData"=w62, "error in (no error)"=w61) -> ()  [unwired: 1 in, 16 out]
          }
          frame "Init" {
            n16 = local write "localVariables"(w81) -> ()
            n17 = local read "Use"() -> (w84:bool)
            n18 = call <resource>:"UMLEditor getDiagramInfo.vi"("localVariables"=w81, "error in (no error)"=w95) -> ("graph"=w91:refnum<class "Graph.lvclass">, "name"=w87:string, "diagramType"=w94:T33, "saveDir"=w78:path, "error out"=w90:errorcluster)  [unwired: 13 out]
            n19 = case shown="False" w84 {
              frame True {
                n20 = property on="ClassFolderSuffix" class="Str"("Disabled"=u8 0) -> ()  [unwired: 2 in, 2 out]
              }
              frame False {
                n21 = property on="ClassFolderSuffix" class="Str"("Disabled"=u8 2) -> ()  [unwired: 2 in, 2 out]
              }
            }
            n22 = property on="Class creation progress" class="LstBox (strict)"("Item Names"=string[] []) -> ()  [unwired: 2 in, 2 out]
            n23 = property on="Tab" class="TabCtl (strict)"("Value"=enum32{"Create", "Config"}."Create" ("Tab")) -> ()  [unwired: 2 in, 2 out]
            n24 = Empty String/Path?(string/path=w78) -> (empty?=w82:bool)
            n25 = case shown="\"ClassDiagramGraph\"" w94 {
              tunnel: ["GetNodesEdges" "Exit"] -> w93
              frame "ClassDiagramGraph" {
              }
              frame Default {
                n26 = One Button Dialog(message="Classes could only be built from a class diagram!") -> ()  [unwired: 2 out]
              }
            }
            n27 = Not(x=w82) -> (.not. x?=w85:bool)
            n28 = Match Pattern(string=w87, regular expression="[.][~.]+$") -> (before substring=w88:string)  [unwired: 4 out]
            n29 = case shown="False" w82 {
              tunnel: w78 -> [w103 _]
              frame False {
                n30 = local write "ClassPath"(w103) -> ()
              }
              frame True {
              }
            }
            n31 = call <resource>:"File_ApplicationPaths.vi"("PathName"=UMLEditor_StoredPathes."ClassBasePath" ("UMLPathes")) -> ("Path Out"=w79:path)  [unwired: 3 in, 15 out]
            n32 = Concatenate Strings(w88, ".txt" ("string")) -> (w76:string)
            n33 = Select(t=w78, s=w85, f=w79) -> (s? t:f=w77:path)
            n34 = call <resource>:"BaseProvider_IniFileSettings.vi"() -> ("IniFileSettings"=w67:T34)  [unwired: 18 in, 1 out]
            n35 = Build Path(base path=w77, name or relative path=w76) -> (appended path=w75:path)
            n36 = Unbundle By Name(w67) -> ("ClassFolderSuffix"=w66:string, "InterfaceFolderSuffix"=w65:string)
            n37 = Empty String/Path?(string/path=w77) -> (empty?=w83:bool)
            n38 = case shown="False" w83 {
              tunnel: w75 -> [w96 _]
              frame False {
                n39 = local write "ScriptfilePath"(w96) -> ()
              }
              frame True {
                n40 = local read "ScriptfilePath"() -> (w98:path)
                n41 = call <resource>:"GOOP_GetGDSConfigFolder.vi"() -> ("GDSFolderPath"=w102:path)
                n42 = Empty String/Path?(string/path=w98) -> (empty?=w100:bool)
                n43 = Build Path(base path=w102, name or relative path="Testscript.txt") -> (appended path=w99:path)
                n44 = Select(t=w99, s=w100, f=w98) -> (s? t:f=w97:path)
                n45 = local write "ScriptfilePath"(w97) -> ()
              }
            }
            n46 = property on="Class creation progress" class="LstBox (strict)"("Top Row"=0) -> ()  [unwired: 2 in, 2 out]
            n47 = Bundle By Name(cluster=w70, "graph"=w91) -> (w92:T16)
            n48 = call <resource>:"BaseProvider_ConfigurationMemory.vi"("Action"=enum16{"Read", "Load", "Save", "Set"}."Read") -> ("PatternOut"=w68:T1)  [unwired: 12 in, 6 out]
            n49 = local write "ClassFolderSuffix"(w66) -> ()
            n50 = local write "InterfaceFolderSuffix"(w65) -> ()
            n51 = local write "Connector Pane Pattern"(w68) -> ()
            "Class creation progress" <- -1 ("Class creation progress")
          }
          frame "GetNodesEdges" {
            w114 = refnum<class "ClassNode.lvclass"> refnum ("reference")
            w116 = refnum<class "ClassNode.lvclass">[] [] ("nodes")
            n52 = Unbundle By Name(w119) -> ("SelectedNodes"=w122:refnum<class "AbstractNode.lvclass">[])
            n53 = Unbundle By Name(w126) -> ("graph"=w124:refnum<class "Graph.lvclass">)
            n54 = call-dynamic "getNodes.vi"("reference"=w124, "error in (no error)"=w129) -> ("nodes"=w113:refnum<class "AbstractNode.lvclass">[], "error out"=w133:errorcluster)  [unwired: 15 in, 1 out]
            n55 = Select(t=w122, s=w121, f=w113) -> (s? t:f=w123:refnum<class "AbstractNode.lvclass">[])
            n56 = Index Array(array=w123) -> ()  [unwired: 1 in, 1 out]
            n57 = for {
              shift-right: [w180] -> w132
              shift-left: w133 -> [w182]
              tunnel: w123 -> [w181] mode=indexing
              shift-right: [w177] -> w118
              shift-left: w116 -> [w179]
              n58 = call <resource>:"AbstractNode_GetObjectStatus.vi"("reference in"=w181, "error in (no error)"=w182) -> ("Class name"=w176:string, "reference out"=w178:refnum<class "AbstractNode.lvclass">, "error out"=w180:errorcluster)  [unwired: 15 out]
              n59 = case shown="\"ClassNode\", \"InterfaceNode\"" w176 {
                tunnel: w179 -> [w187 w188]
                tunnel: w178 -> [w185 _]
                tunnel: [w186 w188] -> w177
                frame "ClassNode", "InterfaceNode" {
                  n60 = To More Specific Class(target class=refnum<class "ClassNode.lvclass"> refnum ("reference"), reference=w185) -> (specific class reference=w184:refnum<class "ClassNode.lvclass">)  [unwired: 1 in, 1 out]
                  n61 = Build Array (concatenate)(w187, w184) -> (w186:refnum<class "ClassNode.lvclass">[])
                }
                frame Default {
                }
              }
            }
            n62 = for {
              tunnel: w113 -> [w135] mode=indexing
              tunnel: [w134] -> w112 mode=indexing
              n63 = To More Specific Class(target class=refnum<class "ClassNode.lvclass"> refnum ("reference"), reference=w135) -> (specific class reference=w134:refnum<class "ClassNode.lvclass">)  [unwired: 1 in, 1 out]
            }
            n64 = call-dynamic "getEdges.vi"("reference"=w124, "error in (no error)"=w132) -> ("edges"=w130:refnum<class "AbstractEdge.lvclass">[], "error out"=w131:errorcluster)  [unwired: 15 in, 1 out]
            n65 = for {
              shift-right: [w150] -> w128
              shift-left: w131 -> [w155]
              tunnel: w130 -> [w154] mode=indexing
              shift-right: [w152] -> w125
              shift-left: w116 -> [w153]
              shift-right: [w148] -> w120
              shift-left: w116 -> [w147]
              tunnel: refnum<class "ClassRelationshipEdge.lvclass"> refnum ("nodeRef") -> [w144]
              tunnel: w114 -> [w142]
              tunnel: w114 -> [w141]
              tunnel: [w138] -> w111 mode=indexing if=w140
              tunnel: [w138] -> w110 mode=indexing if=w139
              tunnel: [w138] -> w109 mode=indexing if=w137
              n66 = call-dynamic "isInheritance.vi"("reference"=w154, "error in (no error)"=w155) -> ("reference out"=w143:refnum<class "AbstractEdge.lvclass">, "isInheritance"=w140:bool, "isCompAggregation"=w139:bool, "isInterfaecImplementing"=w137:bool, "error out"=w151:errorcluster)  [unwired: 13 in]
              n67 = To More Specific Class(target class=w144, reference=w143) -> (specific class reference=w138:refnum<class "ClassRelationshipEdge.lvclass">)  [unwired: 1 in, 1 out]
              n68 = case shown="True" w140 {
                tunnel: w151 -> [w168 w175]
                tunnel: [w168 w174] -> w150
                tunnel: w138 -> [_ w173]
                tunnel: [FALSE ("inheritanceUsed") w172] -> w146
                tunnel: [_ w171] -> w149
                tunnel: [_ w170] -> w145
                frame False {
                }
                frame True {
                  n69 = call <resource>:"WhoInheritsWhom.vi"("reference"=w173, "error in (no error)"=w175) -> ("inherits"=w171:refnum<class "AbstractNode.lvclass">, "base"=w170:refnum<class "AbstractNode.lvclass">, "inheritanceUsed"=w172:bool, "error out"=w174:errorcluster)  [unwired: 14 out]
                }
              }
              n70 = case shown="True" w146 {
                tunnel: w145 -> [_ w159]
                tunnel: w147 -> [w156 w161]
                tunnel: [w156 w160] -> w148
                tunnel: w142 -> [_ w157]
                frame False {
                }
                frame True {
                  n71 = To More Specific Class(target class=w157, reference=w159) -> (specific class reference=w158:refnum<class "ClassNode.lvclass">)  [unwired: 1 in, 1 out]
                  n72 = Build Array (concatenate)(w161, w158) -> (w160:refnum<class "ClassNode.lvclass">[])
                }
              }
              n73 = case shown="True" w146 {
                tunnel: w149 -> [_ w165]
                tunnel: w153 -> [w162 w167]
                tunnel: [w162 w166] -> w152
                tunnel: w141 -> [_ w163]
                frame False {
                }
                frame True {
                  n74 = To More Specific Class(target class=w163, reference=w165) -> (specific class reference=w164:refnum<class "ClassNode.lvclass">)  [unwired: 1 in, 1 out]
                  n75 = Build Array (concatenate)(w167, w164) -> (w166:refnum<class "ClassNode.lvclass">[])
                }
              }
            }
            n76 = Bundle By Name(cluster=w126, "AllNodes"=w112, "nodes"=w118, "baseNodes"=w120, "subNodes"=w125, "InheritEdges"=w111, "CompAggEdges"=w110, "InterfaceEdges"=w109) -> (w127:T16)
          }
          frame "GetClassData" {
            n77 = Unbundle By Name(w202) -> ("subNodes"=w194:refnum<class "ClassNode.lvclass">[], "classes"=w205:T15[])  [unwired: 1 out]
            n78 = Unbundle By Name(w202) -> ("nodes"=w206:refnum<class "ClassNode.lvclass">[])
            n79 = Index Array(array=w205) -> (element=w203:T15)  [unwired: 1 in]
            n80 = Index Array(array=w206) -> (element=w197:refnum<class "ClassNode.lvclass">)  [unwired: 1 in]
            n81 = Initialize Array(w203, 0 ("dimension size")) -> (w190:T15[])
            n82 = Initialize Array(w197, 0 ("dimension size")) -> (w193:refnum<class "ClassNode.lvclass">[])
            n83 = for {
              tunnel: w206 -> [w210] mode=indexing
              shift-right: [w238] -> w191
              shift-left: w190 -> [w220]
              tunnel: w199 -> [w237]
              shift-right: [w235] -> w198
              shift-left: w200 -> [w236]
              tunnel: w199 -> [w234]
              shift-right: [w230] -> w195
              shift-left: w193 -> [w229]
              tunnel: w194 -> [w228]
              shift-right: [w224] -> w192
              shift-left: w193 -> [w225]
              w211 = refnum<class "InterfaceNode.lvclass"> refnum  # InterfaceNode.lvclass
              n84 = call-dynamic "getClassInfo.vi"("reference"=w210, "error in (no error)"=w236) -> ("className"=w223:string, "methods"=w227:string[], "ClassPath"=w226:path, "error out"=w235:errorcluster)  [unwired: 8 in, 6 out]
              n85 = To More Specific Class(target class=w211, reference=w210) -> (error out=w209:errorcluster)  [unwired: 1 in, 1 out]
              n86 = Unbundle By Name(w209) -> ("status"=w208:bool)
              n87 = call <resource>:"CommonVIs SterotypeStringParser.vi"("SterotypeStringIn"=w223) -> ("StereoType"=w221:T36, "Name"=w217:string, "Sterotype"=w222:string)  [unwired: 16 out]
              n88 = for {
                tunnel: w220 -> [w240] mode=indexing
                tunnel: [w239] -> w219 mode=indexing
                n89 = Unbundle By Name(w240) -> ("ClassName"=w239:string)
              }
              n90 = To Lower Case(string=w217) -> (all lower case string=w216:string)
              n91 = To Lower Case(string=w219) -> (all lower case string=w218:string[])
              n92 = Not(x=w208) -> (.not. x?=w207:bool)
              n93 = Empty String/Path?(string/path=w223) -> (empty?=w214:bool)
              n94 = Search 1D Array(1D array=w218, element=w216) -> (index of element=w213:i32)  [unwired: 1 out]
              n95 = Greater Or Equal To 0?(x=w213) -> (x >= 0?=w212:bool)
              n96 = Or(x=w214, y=w212) -> (x .or. y?=w215:bool)
              n97 = Unbundle By Name(w234) -> ("Methods"=w233:T37)
              n98 = Index Array(array=w233) -> (element=w232:T38)  [unwired: 1 in]
              n99 = for {
                tunnel: w227 -> [w320] mode=indexing
                tunnel: w232 -> [w319]
                tunnel: [w318] -> w231 mode=indexing
                n100 = Match Pattern(string=w320, regular expression="<[~>]+[>]+") -> (before substring=w300:string, after substring=w301:string, offset past match=w302:i32)  [unwired: 2 out]
                n101 = Less Than 0?(x=w302) -> (x < 0?=w303:bool)
                n102 = Select(t=w300, s=w303, f=w301) -> (s? t:f=w299:string)
                n103 = call <resource>:"CommonVIs RemoveWhiteSpace.vi"("Remove from"=enum16{"Begining", "End", "Beg+End", "All"}."All", "String in"=w299) -> ("String out"=w317:string)  [unwired: 2 in, 3 out]
                n104 = Match Pattern(string=w317, regular expression="^[+-#]") -> (before substring=w315:string, match substring=w298:string, after substring=w314:string)  [unwired: 2 out]
                n105 = Concatenate Strings(w315, w314) -> (w306:string)
                n106 = Equal?(x=w298, y="-") -> (x = y?=w312:bool)
                n107 = Equal?(x=w298, y="#") -> (x = y?=w296:bool)
                n108 = Match Pattern(string=w306, regular expression="(") -> (before substring=w304:string)  [unwired: 4 out]
                n109 = for {
                  tunnel: [w325] -> w311 mode=indexing
                  tunnel: w304 -> [w324]
                  tunnel: string[] ["^[gG][eE][tT]", "^[cC][hH][eE][cC][kK]", "^[rR][eE][aA][dD]"] -> [w323] mode=indexing
                  n110 = Match Pattern(string=w324, regular expression=w323) -> (offset past match=w326:i32)  [unwired: 4 out]
                  n111 = Greater Or Equal To 0?(x=w326) -> (x >= 0?=w325:bool)
                }
                n112 = Or Array Elements(Boolean array=w311) -> (logical OR=w310:bool)
                n113 = Not(x=w310) -> (.not. x?=w309:bool)
                n114 = Boolean To (0,1)(Boolean=w309) -> (0, 1=w308:i16)
                n115 = Bundle By Name(cluster=w319, "MethodName"=w304, "Private"=w312, "Protected"=w296, "Method Type"=w308) -> (w318:T38)
              }
              n116 = case shown="False" w215 {
                tunnel: w220 -> [w255 w294]
                tunnel: [w254 w294] -> w238
                tunnel: w237 -> [w253 _]
                tunnel: w231 -> [w252 _]
                tunnel: [w251 w295] -> w230
                tunnel: w229 -> [w250 w295]
                tunnel: w210 -> [w249 _]
                tunnel: w228 -> [w248 _]
                tunnel: w226 -> [w247 _]
                tunnel: w225 -> [w246 w293]
                tunnel: [w245 w293] -> w224
                tunnel: w217 -> [w244 _]
                tunnel: w222 -> [w243 _]
                tunnel: w221 -> [w242 _]
                tunnel: w207 -> [w241 _]
                frame False {
                  n117 = case shown="Default" w242 {
                    tunnel: w255 -> [w280 w289 w291]
                    tunnel: [w279 w289 w291] -> w254
                    tunnel: w244 -> [w264 _ _]
                    tunnel: w253 -> [w276 _ _]
                    tunnel: w252 -> [w277 _ _]
                    tunnel: [w275 w288 w292] -> w251
                    tunnel: w250 -> [w274 w288 w292]
                    tunnel: w249 -> [w269 w285 _]
                    tunnel: w248 -> [w272 _ _]
                    tunnel: w247 -> [w262 _ _]
                    tunnel: w243 -> [w268 _ _]
                    tunnel: w246 -> [w270 w287 w290]
                    tunnel: [w270 w286 w290] -> w245
                    tunnel: w241 -> [w256 _ _]
                    frame Default {
                      n118 = Search 1D Array(1D array=w272, element=w269) -> (index of element=w271:i32)  [unwired: 1 out]
                      n119 = call <vilib>:"Get File Extension.vi"("file"=w262) -> ("lowercase file extension"=w267:string)  [unwired: 1 in, 9 out]
                      n120 = Greater Or Equal To 0?(x=w271) -> (x >= 0?=w258:bool)
                      n121 = Boolean To (0,1)(Boolean=w258) -> (0, 1=w273:i16)
                      n122 = Concatenate Strings(w264, ".lvclass" ("string")) -> (w265:string)
                      n123 = case shown="\"lvclass\"" w267 {
                        tunnel: w262 -> [w283 w284]
                        tunnel: [w282 w284] -> w266
                        tunnel: w265 -> [w281 _]
                        frame Default {
                          n124 = Build Path(base path=w283, name or relative path=w281) -> (appended path=w282:path)
                        }
                        frame "lvclass" {
                        }
                      }
                      n125 = Not(x=w258) -> (.not. x?=w257:bool)
                      n126 = call <resource>:"Common_DoesClassExist.vi"("ClassPath"=w266, "ClassName"=w264) -> ("ClassExists"=w261:bool)  [unwired: 17 out]
                      n127 = Empty String/Path?(string/path=w262) -> (empty?=w259:bool)
                      n128 = Compound Arithmetic op=AND(invert w259, w261) -> (w260:bool)
                      n129 = Bundle By Name(cluster=w276, "Node"=w269, "BaseClass"=w257, "ClassType"=w273, "ClassName"=w264, "Class folder"=w262, "ClassStereotype"=w268, "ExistsAsFile"=w260, "Methods"=w277, "Interface"=w256) -> (w278:T15)
                      n130 = Build Array (concatenate)(w274, w269) -> (w275:refnum<class "ClassNode.lvclass">[])
                      n131 = Build Array (concatenate)(w280, w278) -> (w279:T15[])
                    }
                    frame "TYPE", "ENUM" {
                      n132 = Build Array (concatenate)(w287, w285) -> (w286:refnum<class "ClassNode.lvclass">[])
                    }
                    frame "APPLICATION".."LVLIB" {
                    }
                  }
                }
                frame True {
                }
              }
            }
            n133 = Bundle By Name(cluster=w202, "nodes"=w195, "classes"=w191, "Types"=w192) -> (w201:T16)
          }
          frame "GetProviders" {
            (unwired) "Exit" ("y")
            # "Classes to create"
            n134 = Unbundle By Name(w339) -> ("nodes"=w334:refnum<class "ClassNode.lvclass">[], "classes"=w335:T15[])
            n135 = Array Size(array=w335) -> (size(s)=w337:i32)
            n136 = for {
              tunnel: w335 -> [w344] mode=indexing
              tunnel: [w342] -> w338 mode=indexing
              n137 = Unbundle By Name(w344) -> ("ExistsAsFile"=w343:bool)
              n138 = Boolean To (0,1)(Boolean=w343) -> (0, 1=w342:i16)
            }
            n139 = Add Array Elements(numeric array=w338) -> (sum=w333:i16)
            n140 = Subtract(x=w337, y=w333) -> ()  [unwired: 1 out]
            n141 = call <resource>:"GOOP_CurrentProviderClass_Memory.vi"() -> ("AllClassProviders(OriginalNames)"=w329:string[], "ClassProviderName"=w341:string, "AllClassProviders(TranslatedNames)"=w330:string[])  [unwired: 7 in, 10 out]
            n142 = property on="_CurrentClassProvider" class="Ring (strict)"("Strings []"=w330) -> ()  [unwired: 2 in, 2 out]
            n143 = Search 1D Array(1D array=w329, element=w341) -> (index of element=w327:i32)  [unwired: 1 out]
            n144 = Max & Min(x=w327, y=0) -> (max(x,y)=w328:i32)  [unwired: 1 out]
            n145 = Bundle By Name(cluster=w339, "nodes"=w334, "classes"=w335, "Providers"=w329, "ClassProvider"=w327) -> (w340:T16)
            n146 = local write "_CurrentClassProvider"(w328) -> ()
          }
          frame "SetDefaultData" {
            n147 = Unbundle By Name(w363) -> ("classes"=w347:T15[])
            n148 = Tick Count (ms)() -> (millisecond timer value=w355:u32)
            n149 = for {
              tunnel: w347 -> [w366] mode=indexing
              tunnel: [w364] -> w349 mode=indexing
              n150 = Unbundle By Name(w366) -> ("ExistsAsFile"=w365:bool)
              n151 = Boolean To (0,1)(Boolean=w365) -> (0, 1=w364:i16)
            }
            n152 = Array Size(array=w347) -> (size(s)=w348:i32)
            n153 = Array Size(array=w354) -> (size(s)=w357:i32)
            n154 = Add Array Elements(numeric array=w349) -> (sum=w346:i16)
            n155 = Subtract(x=w348, y=w346) -> (x-y=w345:i32)
            n156 = local read "Classes"() -> (w359:T2)
            n157 = Index Array(array=w359) -> (element=w358:T39)  [unwired: 1 in]
            n158 = for {
              tunnel: w347 -> [w398] mode=indexing
              tunnel: [w398] -> w362 mode=indexing
              tunnel: w358 -> [w397]
              tunnel: w357 -> [w390]
              tunnel: w354 -> [w389]
              tunnel: w355 -> [w383]
              tunnel: w353 -> [w377]
              shift-right: [w372] -> w351
              shift-left: T2 [] ("Classes") -> [w368]
              tunnel: w345 -> [w369]
              i -> [w370]
              w375 = u32 16448250
              n159 = Add(x=w383, y=w370) -> (x+y=w384:u32)
              n160 = Unbundle By Name(w398) -> ("ClassName"=w380:string, "ClassType"=w396:i32, "ExistsAsFile"=w373:bool)
              n161 = Array Size(array=w368) -> (size(s)=w367:i32)
              n162 = Quotient & Remainder(x=w384, y=w390) -> (x-y*floor(x/y)=w378:u32)  [unwired: 1 out]
              n163 = Index Array(array=w389, index=w378) -> (element=w388:u32)
              n164 = Increment(x=w367) -> (x+1=w386:i32)
              n165 = Index Array(array=w377, index=w378) -> (element=w376:u32)
              n166 = Equal?(x=w396, y=0) -> (x = y?=w381:bool)
              n167 = Format Into String(format string="%d of %d", w386, w369) -> (resulting string=w385:string)  [unwired: 2 in, 1 out]
              n168 = Select(t=u32 0, s=w381, f=u32 255) -> (s? t:f=w392:u32)
              n169 = call <resource>:"UMLEditor_GenerateShortClassIconName.vi"("ClassName"=w380) -> ("ShortClassIconName"=w379:string)
              n170 = Bundle By Name(cluster=w397, "ClassName"=w380, "Class icon name"=w379, "Frame"=w392, "Header"=w388, "Public"=w376, "Private"=w375, "Protected"=w375, "Text"=u32 0, "text"=w385, "Class description"="", "UseVirtuals"=TRUE, "ClassIdex"=w370) -> (w371:T39)
              n171 = case shown="True" w373 {
                tunnel: [w401 w402] -> w372
                tunnel: w368 -> [w400 w402]
                tunnel: w371 -> [w399 _]
                frame False {
                  n172 = Build Array (concatenate)(w400, w399) -> (w401:T2)
                }
                frame True {
                }
              }
            }
            n173 = Bundle By Name(cluster=w363, "classes"=w362) -> (w361:T16)
            n174 = local write "Classes"(w351) -> ()
            n175 = property on="Classes" class="Arr (strict)"(error in=w350, "Index Values"=u32[] [0]) -> ()  [unwired: 1 in, 2 out]
          }
          frame "ClassPathVisible" {
            n176 = Unbundle By Name(w405) -> ("classes"=w410:T15[])
            n177 = for {
              tunnel: w410 -> [w416] mode=indexing
              tunnel: [w414] -> w409 mode=indexing
              n178 = Unbundle By Name(w416) -> ("Class folder"=w415:path)
              n179 = Empty String/Path?(string/path=w415) -> (empty?=w414:bool)
            }
            n180 = Or Array Elements(Boolean array=w409) -> (logical OR=w408:bool)
            n181 = Select(t=u8 0 ("Disabled"), s=w408, f=u8 2) -> (s? t:f=w406:u8)
            n182 = property on="ClassPath" class="Path"("Disabled"=w406) -> ()  [unwired: 2 in, 2 out]
            n183 = local read "ScriptfilePath"() -> (w403:path)
            n184 = property on="ClassFolderSuffix" class="Str"("Disabled"=w406) -> ()  [unwired: 2 in, 2 out]
            n185 = Bundle By Name(cluster=w405, "scriptFilePath"=w403) -> (w404:T16)
          }
          frame "CheckProject" {
            n186 = call <resource>:"CommonVIs_UmlOpenVIRef.vi"("error in"=w424) -> ("error out"=w430:errorcluster, "ProjectNameOut"=w419:string)  [unwired: 3 in, 6 out]
            n187 = call <resource>:"GDSProject_GetProjects.vi"("GetProjectRefByName"=w419, "error in (no error)"=w430) -> ("Projects"=w421:string[], "Project Refnum"=w418:refnum<vi>, "error out"=w423:errorcluster)  [unwired: 1 in, 14 out]
            n188 = Search 1D Array(1D array=w421, element=w419) -> (index of element=w429:i32)  [unwired: 1 out]
            n189 = Max & Min(x=w429, y=0) -> (max(x,y)=w420:i32)  [unwired: 1 out]
            n190 = Index Array(array=w421, index=w420) -> (element=w427:string)
            n191 = Empty String/Path?(string/path=w427) -> (empty?=w426:bool)
            n192 = case shown="True" w426 {
              tunnel: ["Modify?" w445] -> w425
              tunnel: w423 -> [w439 w446]
              tunnel: [w439 w446] -> w422
              tunnel: w421 -> [w438 _]
              tunnel: w420 -> [w437 _]
              tunnel: w418 -> [w436 w442]
              tunnel: [w432 _] -> _
              frame False {
                n193 = local write "Project"(w437) -> ()
                n194 = property on="Project" class="Ring (strict)"("Strings []"=w438) -> ()  [unwired: 2 in, 2 out]
                n195 = property class="Project"(reference=w436) -> (reference out=w433:refnum<vi>, error out=w431:errorcluster, "Path"=w434:path)  [unwired: 1 in]
                n196 = Strip Path(path=w434) -> (stripped path=w435:path)  [unwired: 1 out]
                n197 = Close Reference(reference=w433, error in (no error)=w431) -> (error out=w432:errorcluster)
                n198 = local write "ClassPath"(w435) -> ()
              }
              frame True {
                n199 = Close Reference(reference=w442) -> (error out=w441:errorcluster)  [unwired: 1 in]
                n200 = File Dialog(4:"LabVIEW projects" ("pattern label"), 5:"Open" ("button label"), 6:"*.lvproj" ("pattern (all files)"), 7:"Select a project to open" ("prompt")) -> (1:w447:bool, 3:w444:path)  [unwired: 3 in, 2 out]
                n201 = case shown="False" w447 {
                  tunnel: w444 -> [w463 _]
                  tunnel: ["Modify?" "Exit" ("y")] -> w445
                  tunnel: w441 -> [_ _]
                  frame False {
                    n202 = call <vilib>:"Set Busy.vi"() -> ("error out"=w457:errorcluster)  [unwired: 4 in, 7 out]
                    n203 = invoke class="App" method="Project.Open"(error in=w457, "Path"=w463) -> ("Project:Open"=w462:refnum<vi>)  [unwired: 2 in, 3 out]
                    n204 = invoke class="Project" method="Open Window"(reference=w462) -> (reference out=w460:refnum<vi>, error out=w461:errorcluster)  [unwired: 2 in, 1 out]
                    n205 = Close Reference(reference=w460, error in (no error)=w461) -> (error out=w459:errorcluster)
                    n206 = call <resource>:"GDSProject_GetProjects.vi"("error in (no error)"=w459) -> ("Projects"=w458:string[])  [unwired: 2 in, 16 out]
                    n207 = Index Array(array=w458) -> (element=w453:string)  [unwired: 1 in]
                    n208 = call <resource>:"GDSProject_GetProjects.vi"("GetProjectRefByName"=w453) -> ("Projects"=w455:string[])  [unwired: 2 in, 16 out]
                    n209 = call <resource>:"UMLEditor_TargetDialog.vi"("SetLastSearchPath(True)"=FALSE, "GetProjectRefByName"=w453) -> ()  [unwired: 5 in, 5 out]
                    n210 = property on="Project" class="Ring (strict)"("Strings []"=w455) -> ()  [unwired: 2 in, 2 out]
                    n211 = local write "Project"(0) -> ()
                    n212 = call <vilib>:"Unset Busy.vi"() -> ()  [unwired: 2 in, 10 out]
                  }
                  frame True {
                  }
                }
                n213 = Strip Path(path=w444) -> (stripped path=w443:path)  [unwired: 1 out]
                n214 = local write "ClassPath"(w443) -> ()
              }
            }
          }
          frame "Modify?" {
            n215 = Unbundle By Name(w466) -> ("Types"=w468:refnum<class "ClassNode.lvclass">[], "classes"=w471:T15[])
            n216 = Array Size(array=w471) -> (size(s)=w469:i32)
            n217 = case shown="1.." w469 {
              selector: w469 -> [_ w536]
              tunnel: w468 -> [w476 _]
              tunnel: [w474 w522] -> w465
              tunnel: w466 -> [w473 w524]
              tunnel: [w472 w527] -> w467
              tunnel: w466 -> [_ w525]
              frame 0, Default {
                n218 = Array Size(array=w476) -> (size(s)=w475:i32)
                n219 = case shown="1.." w475 {
                  tunnel: [w482 "Exit" ("t")] -> w474
                  tunnel: w473 -> [w481 w517]
                  tunnel: [w480 w518] -> w472
                  frame 1.. {
                    n220 = local read "ClassPath"() -> (w484:path)
                    n221 = Format Into String(format string="Only Types where found.\nDo you want to create these types in this directory:\n%s\n(If ClassPath defined that path will be used)" ("message"), w484) -> (resulting string=w488:string)  [unwired: 2 in, 1 out]
                    n222 = call <resource>:"GOOP_GetGDSConfigFolder.vi"() -> ("GDSFolderPath"=w479:path)
                    n223 = Build Path(base path=w479, name or relative path="Testscript.txt") -> (appended path=w477:path)
                    n224 = call <vilib>:"Three Button Dialog.vi"("Right Button Text (\"Cancel\")"="Cancel" ("Right Button Text (\"Cancel\")"), "Center Button Text (\"No\")"="Change directory" ("Center Button Text (\"No\")"), "Left Button Text (\"Yes\")"="Create here" ("Left Button Text (\"Yes\")"), "message"=w488) -> ("Which Button?"=w483:T40)  [unwired: 1 in, 6 out]
                    n225 = case shown="\"Center Button\"" w483 {
                      tunnel: ["CreateTypeDefs" ("y") w499 "Exit" ("t")] -> w482
                      tunnel: w481 -> [w494 w498 w513]
                      tunnel: [w493 w497 w514] -> w480
                      tunnel: w477 -> [w492 w496 _]
                      frame "Left Button", Default {
                        n226 = Delete(path (use dialog)=w492) -> (deleted path=w491:path)  [unwired: 1 in, 5 out]
                        n227 = Bundle By Name(cluster=w494, "cancel"=FALSE, "scriptFilePath"=w491) -> (w493:T16)
                      }
                      frame "Center Button" {
                        (unwired) T41."existing dir" ("select mode (2)")
                        n228 = File Dialog() -> (1:w501:bool, 3:w500:path)  [unwired: 1 in, 8 out]
                        n229 = case shown="False" w501 {
                          tunnel: w500 -> [w508 _]
                          tunnel: ["CreateTypeDefs" ("y") "Exit" ("t")] -> w499
                          tunnel: w498 -> [w505 w511]
                          tunnel: [w504 w510] -> w497
                          tunnel: w496 -> [w502 _]
                          frame False {
                            n230 = Delete(path (use dialog)=w502) -> (deleted path=w503:path)  [unwired: 1 in, 5 out]
                            n231 = local write "ClassPath"(w508) -> ()
                            n232 = Bundle By Name(cluster=w505, "cancel"=FALSE, "scriptFilePath"=w503) -> (w504:T16)
                          }
                          frame True {
                            n233 = Bundle By Name(cluster=w511, "cancel"=TRUE) -> (w510:T16)
                          }
                        }
                      }
                      frame "Right Button" {
                        n234 = Bundle By Name(cluster=w513, "cancel"=TRUE) -> (w514:T16)
                      }
                    }
                  }
                  frame Default {
                    n235 = One Button Dialog(message="Sorry!\nCould not find any classes to create script from.\nAll classes with names could be created,\nbut you haven't any classes with names yet.") -> ()  [unwired: 2 out]
                    n236 = Bundle By Name(cluster=w517, "cancel"=TRUE) -> (w518:T16)
                  }
                }
              }
              frame 1.. {
                n237 = call <resource>:"CommonVIs_GetFrontPanelControls.vi"() -> ("Event Registration Refnum"=w534:refnum<event-registration>, "ControlRefs"=w535:refnum<vi>[])  [unwired: 2 in, 16 out]
                n238 = while {
                  tunnel: [w549] -> w526
                  tunnel: [w548] -> w528
                  tunnel: w536 -> [w550]
                  shift-right: [w544] -> w533
                  shift-left: w534 -> [w545]
                  tunnel: w525 -> [w540]
                  shift-right: [w537] -> w523
                  shift-left: w524 -> [w538]
                  stop <- w547 stop-if-true
                  n239 = Unbundle By Name(w540) -> ("Providers"=w539:string[])
                  n240 = local read "_CurrentClassProvider"() -> (w541:u16)
                  n241 = event shown="[6] \"_CurrentClassProvider\": Value Change" {
                    selector: w545 -> [_ _ _ _ _ _ _ _ _ _ _ _ _]
                    dyn-events: [_ _ _ _ _ _ _ _ _ _ _ _ _] -> w544
                    timeout: 500 -> [_ _ _ _ _ _ _ _ _ _ _ _ _]
                    tunnel: w550 -> [_ _ _ _ _ _ _ _ w588 _ _ _ _]
                    tunnel: [_ _ _ TRUE ("Cancel") _ _ _ _ _ _ _ _ "Cancel 2"] -> w549
                    tunnel: [_ _ _ _ _ _ _ _ _ "CreateClasses" _ _ _] -> w548
                    tunnel: w538 -> [w558 w560 w566 w569 w571 w576 w580 w581 w587 w600 w606 w615 w621]
                    tunnel: [w558 w560 w566 w569 w571 w576 w580 w581 w587 w600 w605 w615 w621] -> w537
                    event Timeout {
                      n242 = event-data() -> ()  [unwired: 2 out]
                      n243 = property class="VI"("Front Panel Window:Is Frontmost"=TRUE) -> ()  [unwired: 2 in, 2 out]
                    }
                    event "Help": Value Change {
                      n244 = event-data() -> ()  [unwired: 2 out]
                      n245 = case shown="False" "Help" {
                        tunnel: [ContextHelp_HelpTexts."None(Hide)" ("HelpText") ContextHelp_HelpTexts."UMLEditor createWizardScriptFile_Help" ("HelpText")] -> w562
                        frame False {
                        }
                        frame True {
                        }
                      }
                      n246 = call <resource>:"ContextHelp_HelpTexts.vi"("HelpText (enum or string)"=w562) -> ("HelpOut"=w563:T42)  [unwired: 18 out]
                      n247 = call <resource>:"ContextHelp_SendMessageToPopUp.vi"("PopUpMessage"=w563) -> ()  [unwired: 2 in, 17 out]
                    }
                    event Mouse Enter {
                      n248 = event-data() -> ("CtlRef"=w568:refnum<vi>)  [unwired: 1 out]
                      n249 = local read "Help"() -> (w567:bool)
                      n250 = call <resource>:"ContextHelp_CheckHelpForControl.vi"("Ctl Refnum"=w568, "Help"=w567) -> ()  [unwired: 1 in, 17 out]
                    }
                    event Panel Close {
                      n251 = event-data() -> ()  [unwired: 5 out]
                    }
                    event "Project": Value Change {
                      n252 = event-data() -> ()  [unwired: 7 out]
                      n253 = property on="Project" class="Ring (strict)"() -> ("Strings []"=w575:string[])  [unwired: 2 in, 2 out]
                      n254 = Index Array(array=w575, index="Project") -> (element=w573:string)
                      n255 = call <resource>:"UMLEditor_TargetDialog.vi"("GetProjectRefByName"=w573) -> ("ProjectFolder"=w572:path)  [unwired: 6 in, 4 out]
                      n256 = local write "ClassPath"(w572) -> ()
                    }
                    event "_UseLLB": Value Change {
                      n257 = event-data() -> ()  [unwired: 7 out]
                    }
                    event "_CurrentClassProvider": Value Change {
                      n258 = event-data() -> ()  [unwired: 4 out]
                      n259 = Unbundle By Name(w580) -> ("Providers"=w579:string[])
                      n260 = Index Array(array=w579, index="_CurrentClassProvider") -> (element=w577:string)
                      n261 = call <resource>:"GOOP_CurrentProviderClass_Memory.vi"("SetDefaultClassProvider(Ignored if not wired)"=w577) -> ()  [unwired: 12 in, 7 out]
                    }
                    event "Use": Value Change {
                      n262 = event-data() -> ()  [unwired: 6 out]
                      n263 = case shown="True" "Use" {
                        frame True {
                          n264 = property on="ClassPath" class="Path"() -> ("Disabled"=w585:u8)  [unwired: 2 in, 2 out]
                          n265 = Max & Min(x=u8 0 ("Disabled"), y=w585) -> (max(x,y)=w583:u8)  [unwired: 1 out]
                          n266 = property on="ClassFolderSuffix" class="Str"("Disabled"=w583) -> ()  [unwired: 2 in, 2 out]
                        }
                        frame False {
                          n267 = property on="ClassFolderSuffix" class="Str"("Disabled"=u8 2) -> ()  [unwired: 2 in, 2 out]
                        }
                      }
                    }
                    event "up", "down": Value Change {
                      n268 = event-data() -> ()  [unwired: 6 out]
                      n269 = property on="Classes" class="Arr (strict)"() -> ("Index Values"=w595:u32[])  [unwired: 2 in, 2 out]
                      n270 = Select(t=3, s="down", f=-3 ("t")) -> (s? t:f=w594:i32)
                      n271 = Index Array(array=w595) -> (element=w593:u32)  [unwired: 1 in]
                      n272 = Add(x=w594, y=w593) -> (x+y=w591:u32)
                      n273 = In Range and Coerce(upper limit=w588, x=w591, lower limit=0) -> (In Range?=w592:bool)  [unwired: 1 out]
                      n274 = Build Array(w591) -> (w590:u32[])
                      n275 = case shown="True" w592 {
                        tunnel: w590 -> [_ w599]
                        frame False {
                        }
                        frame True {
                          n276 = property on="Classes" class="Arr (strict)"("Index Values"=w599) -> ()  [unwired: 2 in, 2 out]
                        }
                      }
                    }
                    event "CreateClasses": Value Change {
                      n277 = event-data() -> ()  [unwired: 2 out]
                    }
                    event "ModifyProviders": Value Change {
                      n278 = event-data() -> ()  [unwired: 2 out]
                      n279 = call <resource>:"GOOP_ProviderClasses_SortingDialog.vi"() -> ("error out"=w604:errorcluster, "Cancelled"=w603:bool, "FirstProvider"=w602:string)  [unwired: 9 in]
                      n280 = case shown="False" w603 {
                        tunnel: w606 -> [w613 w614]
                        tunnel: [w612 w614] -> w605
                        tunnel: w604 -> [w608 _]
                        tunnel: w602 -> [w607 _]
                        frame False {
                          w609 = 0 ("y")
                          n281 = call <resource>:"GOOP_CurrentProviderClass_Memory.vi"("error in (no error)"=w608, "SetDefaultClassProvider(Ignored if not wired)"=w607) -> ("AllClassProviders(OriginalNames)"=w610:string[], "AllClassProviders(TranslatedNames)"=w611:string[])  [unwired: 5 in, 11 out]
                          n282 = local write "_CurrentClassProvider"(w609) -> ()
                          n283 = property on="_CurrentClassProvider" class="Ring (strict)"("Strings []"=w611) -> ()  [unwired: 2 in, 2 out]
                          n284 = Bundle By Name(cluster=w613, "Providers"=w610, "ClassProvider"=w609) -> (w612:T16)
                        }
                        frame True {
                        }
                      }
                    }
                    event Value Change {
                      n285 = event-data() -> ()  [unwired: 2 out]
                      n286 = call <resource>:"BaseProvider_ConfigurationMemory.vi"("Action"=enum16{"Read", "Load", "Save", "Set"}."Read") -> ("WireConfigurationOut"=w618:T43, "IconOut"=w617:string)  [unwired: 12 in, 5 out]
                      n287 = call <resource>:"BaseProvider_ConfigurationMemory.vi"("WireConfiguration"=w618, "Icon"=w617, "Action"=enum16{"Read", "Load", "Save", "Set"}."Save", "PatternIn"="Connector Pane Pattern") -> ()  [unwired: 9 in, 7 out]
                    }
                    event "Cancel 2": Value Change {
                      n288 = event-data() -> ()  [unwired: 6 out]
                    }
                  }
                  n289 = Index Array(array=w539, index=w541) -> (element=w542:string)
                  n290 = case shown="\"EndevoGOOP400\", \"OpenG100\"" w542 {
                    tunnel: [TRUE ("Visible") w556] -> w543
                    frame "False", Default {
                      n291 = local read "_UseLLB"() -> (w551:bool)
                      n292 = Select(t=u8 2 ("Disabled"), s=w551, f=u8 0 ("Disabled")) -> (s? t:f=w554:u8)
                      n293 = property on="ClassFolderSuffix" class="Str"("Disabled"=w554) -> ()  [unwired: 2 in, 2 out]
                    }
                    frame "EndevoGOOP400", "OpenG100" {
                      w556 = FALSE ("Visible")
                      n294 = property on="ClassFolderSuffix" class="Str"("Disabled"=u8 0) -> ()  [unwired: 2 in, 2 out]
                      n295 = local write "_UseLLB"(w556) -> ()
                    }
                  }
                  n296 = property on="_UseLLB" class="Bool (strict)"("Visible"=w543) -> ()  [unwired: 2 in, 2 out]
                  n297 = Or(x=w549, y=w548) -> (x .or. y?=w547:bool)
                }
                n298 = Bundle By Name(cluster=w523, "cancel"=w526) -> (w527:T16)
                n299 = Select(t="CheckClassProvider", s=w528, f="Modify?") -> (s? t:f=w532:string)
                n300 = call <resource>:"CommonVIs_CloseControlRefs.vi"("Event Registration Refnum"=w533, "ControlRefs"=w535) -> ()  [unwired: 1 in, 17 out]
                n301 = Select(t="Exit", s=w526, f=w532) -> (s? t:f=w522:string)
              }
            }
          }
          frame "CheckClassProvider" {
            n302 = local read "_CurrentClassProvider"() -> (w636:u16)
            n303 = call <resource>:"CommonVIs_UmlOpenVIRef.vi"() -> ("AppRefOut"=w635:refnum<vi>)  [unwired: 4 in, 7 out]
            n304 = property on="Project" class="Ring (strict)"() -> ("Strings []"=w647:string[])  [unwired: 2 in, 2 out]
            n305 = local read "Project"() -> (w648:u16)
            n306 = property class="App"(reference=w635) -> (error out=w634:errorcluster, "Project.TargetItem"=w633:refnum<vi>)  [unwired: 1 in, 1 out]
            n307 = Index Array(array=w647, index=w648) -> (element=w646:string)
            n308 = property on="Tab" class="TabCtl (strict)"("Value"=enum32{"Create", "Config"}."Config" ("Tab")) -> ()  [unwired: 2 in, 2 out]
            n309 = Bundle By Name(cluster=w650, "ClassProvider"=w636) -> (w624:T16)
            n310 = Unbundle By Name(w624) -> ("Providers"=w623:string[])
            n311 = Index Array(array=w623, index=w636) -> (element=w626:string)
            n312 = call <resource>:"GOOP_CurrentProviderClass_Memory.vi"("error in (no error)"=w649, "SetDefaultClassProvider(Ignored if not wired)"=w626) -> ("error out"=w645:errorcluster)  [unwired: 5 in, 12 out]
            n313 = case shown="No Error" w634 {
              tunnel: w646 -> [_ w661]
              tunnel: w645 -> [w653 w660]
              tunnel: [w653 w658] -> w641
              tunnel: [w652 w655] -> w640
              tunnel: [_ w654] -> w637
              tunnel: w633 -> [w652 _]
              frame No Error {
              }
              frame Error {
                n314 = call <resource>:"GDSProject_GetProjects.vi"("GetProjectRefByName"=w661, "error in (no error)"=w660) -> ("Project Refnum"=w654:refnum<vi>, "error out"=w659:errorcluster)  [unwired: 1 in, 15 out]
                n315 = property class="Project"(reference=w654, error in=w659) -> (error out=w658:errorcluster, "My Computer"=w657:refnum<vi>)  [unwired: 1 out]
                n316 = To More Generic Class(target class=refnum<vi> refnum ("My Computer"), reference=w657) -> (generic class reference=w655:refnum<vi>)
              }
            }
            n317 = property on="Class creation progress" class="LstBox (strict)"("Item Names"=string[] [], "Top Row"=0) -> ()  [unwired: 2 in, 2 out]
            n318 = Match Pattern(string=w626, regular expression="400") -> (offset past match=w628:i32)  [unwired: 1 in, 3 out]
            n319 = Greater Or Equal To 0?(x=w628) -> (x >= 0?=w625:bool)
            n320 = call <resource>:"GOOP_GetClassProvider.vi"("New Item Parent/Object"=w640, "error in (no error)"=w641, "ProviderClassType"=GOOP_ClassProviderClassType."ClassWriter") -> ("LVClass.Open"=w642:refnum<vi>, "error out"=w639:errorcluster)  [unwired: 1 in, 14 out]
            n321 = call <resource>:"GOOP_GetDefaultInstance.vi"("error in"=w639, "LVClassIn"=w642) -> ("error out"=w629:errorcluster, "ClassWriter.lvclass"=w638:refnum<class "ClassWriter.lvclass">)  [unwired: 8 out]
            n322 = Bundle By Name(cluster=w624, "G4"=w625, "My Computer"=w640, "ClassWriterRef"=w638) -> (w644:T16)
            n323 = Close Reference(reference=w637, error in (no error)=w629) -> ()  [unwired: 1 out]
          }
          frame "UpdatePath&Color" {
            n324 = Unbundle By Name(w677) -> ("classes"=w676:T15[])
            n325 = Empty String/Path?(string/path="ClassPath") -> (empty?=w670:bool)
            n326 = Not A Number/Path/Refnum?(number/path/refnum="ClassPath") -> (NaN/Path/Refnum?=w669:bool)
            n327 = Or(x=w670, y=w669) -> (x .or. y?=w668:bool)
            n328 = call <vilib>:"Dflt Data Dir.vi"() -> ("App:Default Data Directory"=w665:path)
            n329 = Select(t=w665, s=w668, f="ClassPath") -> (s? t:f=w666:path)
            n330 = local read "_UseLLB"() -> (w663:bool)
            n331 = for {
              tunnel: "Classes" -> [w712] mode=indexing
              tunnel: w666 -> [w704]
              tunnel: w663 -> [w685]
              shift-right: [w690] -> w674
              shift-left: w676 -> [w691]
              tunnel: "ClassFolderSuffix" -> [w681]
              tunnel: "InterfaceFolderSuffix" -> [w679]
              # "llb?"
              n332 = Unbundle By Name(w712) -> ("ClassIdex"=w686:i32, "ClassName"=w697:string, "Class icon name"=w711:string, "Frame"=w710:u32, "Header"=w709:u32, "Public"=w708:u32, "Private"=w707:u32, "Text"=w706:u32, "Class description"=w705:string, "UseVirtuals"=w703:bool, "Protected"=w699:u32)
              n333 = Index Array(array=w691, index=w686) -> (element=w688:T15)
              n334 = Unbundle By Name(w688) -> ("Interface"=w682:bool, "Class folder"=w695:path)
              n335 = Empty String/Path?(string/path=w695) -> (empty?=w694:bool)
              n336 = Not A Number/Path/Refnum?(number/path/refnum=w695) -> (NaN/Path/Refnum?=w693:bool)
              n337 = Select(t=w679, s=w682, f=w681) -> (s? t:f=w680:string)
              n338 = Or(x=w694, y=w693) -> (x .or. y?=w692:bool)
              n339 = Select(t=".llb", s=w685, f=w680) -> (s? t:f=w684:string)
              n340 = Concatenate Strings(w697, ".lvclass" ("string")) -> (w696:string)
              n341 = case shown="False" w692 {
                tunnel: [w716 w733] -> w701
                tunnel: w697 -> [w714 w734]
                tunnel: w684 -> [w713 w740]
                tunnel: w704 -> [_ w739]
                tunnel: w685 -> [w720 w738]
                tunnel: w695 -> [w717 _]
                tunnel: [w721 w738] -> w702
                tunnel: [w719 w736] -> w700
                tunnel: w696 -> [w715 w735]
                frame False {
                  n342 = call <vilib>:"Get File Extension.vi"("file"=w717) -> ("lowercase file extension"=w718:string)  [unwired: 1 in, 9 out]
                  n343 = case shown="Default" w718 {
                    tunnel: w717 -> [w724 w731]
                    tunnel: [w730 w731] -> w716
                    tunnel: w715 -> [w729 _]
                    tunnel: w713 -> [w728 _]
                    frame Default {
                      n344 = Strip Path(path=w724) -> (stripped path=w725:path, name=w723:string)
                      n345 = Concatenate Strings(w723, w728) -> (w727:string)
                      n346 = Build Path(base path=w725, name or relative path=w727) -> (appended path=w726:path)
                      n347 = Build Path(base path=w726, name or relative path=w729) -> (appended path=w730:path)
                    }
                    frame "lvclass" {
                    }
                  }
                  n348 = call <resource>:"Common_DoesClassExist.vi"("ClassPath"=w716, "ClassName"=w714) -> ("ClassExists"=w719:bool, "llb-class"=w722:bool)  [unwired: 16 out]
                  n349 = Select(t=w722, s=w719, f=w720) -> (s? t:f=w721:bool)
                }
                frame True {
                  n350 = Concatenate Strings(w734, w740) -> (w732:string)
                  n351 = Build Path(base path=w739, name or relative path=w732) -> (appended path=w737:path)
                  n352 = Build Path(base path=w737, name or relative path=w735) -> (appended path=w733:path)
                  n353 = call <resource>:"Common_DoesClassExist.vi"("ClassPath"=w733, "ClassName"=w734) -> ("ClassExists"=w736:bool)  [unwired: 17 out]
                }
              }
              n354 = call <resource>:"UMLEditor_RelativePath.vi"("Path In"=w701) -> ("ConvertToAbsolutePath(If possible)"=w687:path)  [unwired: 1 in, 17 out]
              n355 = Bundle By Name(cluster=w688, "ExistsAsFile"=w700, "LLB"=w702, "Class folder"=w687, "ClassName"=w697, "ClassIconInfo.Icon class name"=w711, "ClassIconInfo.Frame color"=w710, "ClassIconInfo.Header color"=w709, "ClassIconInfo.Public color"=w708, "ClassIconInfo.Private color"=w707, "ClassIconInfo.Foreground color"=w706, "Class description"=w705, "VirtualMethods"=w703, "ClassIconInfo.Protected color"=w699) -> (w689:T15)
              n356 = Replace Array Subset(array=w691, new element=w689, index=w686) -> (w690:T15[])
            }
            n357 = Bundle By Name(cluster=w677, "scriptFilePath"="ScriptfilePath", "classes"=w674) -> (w678:T16)
          }
          frame "UpdateBaseClasses" {
            # "Make sure The Base Class Is added even if not that Node is in the selected \"nodes\"."
            n358 = Unbundle By Name(w754) -> ("InheritEdges"=w755:refnum<class "ClassRelationshipEdge.lvclass">[])
            n359 = Unbundle By Name(w754) -> ("AllNodes"=w746:refnum<class "ClassNode.lvclass">[], "classes"=w752:T15[], "nodes"=w749:refnum<class "ClassNode.lvclass">[])
            n360 = local read "Use"() -> (w747:bool)
            n361 = for {
              tunnel: w755 -> [w781] mode=indexing
              shift-right: [w782] -> w748
              shift-left: w752 -> [w783]
              shift-right: [w779] -> w750
              shift-left: w751 -> [w780]
              tunnel: w749 -> [w760]
              tunnel: w747 -> [w774]
              tunnel: w746 -> [w764]
              tunnel: w745 -> [w773]
              tunnel: [w761] -> w741
              stop <- w761 stop-if-true
              w770 = refnum<class "ClassNode.lvclass"> refnum ("reference")
              n362 = call <resource>:"WhoInheritsWhom.vi"("reference"=w781, "error in (no error)"=w780) -> ("inherits"=w772:refnum<class "AbstractNode.lvclass">, "base"=w771:refnum<class "AbstractNode.lvclass">, "inheritanceUsed"=w763:bool, "error out"=w779:errorcluster)  [unwired: 14 out]
              n363 = To More Specific Class(target class=w770, reference=w772) -> (specific class reference=w769:refnum<class "ClassNode.lvclass">)  [unwired: 1 in, 1 out]
              n364 = To More Specific Class(target class=w770, reference=w771) -> (specific class reference=w759:refnum<class "ClassNode.lvclass">)  [unwired: 1 in, 1 out]
              n365 = call-dynamic "getClassInfo.vi"("reference"=w759) -> ("className"=w767:string, "methods"=w765:string[])  [unwired: 9 in, 8 out]
              n366 = call-dynamic "getClassInfo.vi"("reference"=w769) -> ("className"=w768:string, "ClassPath"=w766:path)  [unwired: 9 in, 8 out]
              n367 = Search 1D Array(1D array=w760, element=w769) -> (index of element=w777:i32)  [unwired: 1 out]
              n368 = Search 1D Array(1D array=w764, element=w759) -> (index of element=w778:i32)  [unwired: 1 out]
              n369 = Search 1D Array(1D array=w760, element=w759) -> (index of element=w758:i32)  [unwired: 1 out]
              n370 = Greater Or Equal To 0?(x=w778) -> (x >= 0?=w775:bool)
              n371 = Greater Or Equal To 0?(x=w777) -> (x >= 0?=w776:bool)
              n372 = Compound Arithmetic op=AND(w776, w775, w763) -> (w762:bool)
              n373 = case shown="True" w762 {
                tunnel: w783 -> [w784 w796]
                tunnel: [w784 w797] -> w782
                tunnel: w777 -> [_ w788]
                tunnel: w778 -> [_ w795]
                tunnel: w774 -> [_ w794]
                tunnel: w759 -> [_ w792]
                tunnel: w773 -> [_ w793]
                tunnel: w764 -> [_ w790]
                tunnel: w768 -> [_ _]
                tunnel: w767 -> [_ _]
                tunnel: w766 -> [_ _]
                tunnel: w765 -> [_ _]
                tunnel: [_ w786] -> w761
                tunnel: w760 -> [_ w789]
                tunnel: w758 -> [_ w785]
                frame False {
                }
                frame True {
                  w791 = 1 items=["Standard class", "Sub class from an existing base class", "Clone class from an existing class"] ("ClassType")
                  n374 = case shown="False" w793 {
                    tunnel: w796 -> [w806 _]
                    tunnel: [w805 w882] -> w787
                    tunnel: w795 -> [w804 _]
                    tunnel: w794 -> [w803 _]
                    tunnel: w792 -> [_ w886]
                    tunnel: w790 -> [w802 _]
                    tunnel: w789 -> [w801 _]
                    tunnel: w785 -> [w800 _]
                    frame False {
                      n375 = disable-structure shown="Enabled" {
                        disable-tunnel: w806 -> [w815 w851 _]
                        disable-tunnel: [w826 w848 w864] -> w805
                        disable-tunnel: w804 -> [w813 w847 w871]
                        disable-tunnel: w803 -> [w824 w845 _]
                        disable-tunnel: w802 -> [w820 _ w872]
                        disable-tunnel: w801 -> [_ _ _]
                        disable-tunnel: w800 -> [w811 _ _]
                        frame Enabled {
                          n376 = Index Array(array=w820, index=w813) -> (element=w819:refnum<class "ClassNode.lvclass">)
                          n377 = Index Array(array=w815, index=w811) -> (element=w814:T15)
                          n378 = Unbundle By Name(w814) -> ("Class folder"=w809:path)
                          n379 = call-dynamic "getClassInfo.vi"("reference"=w819) -> ("className"=w818:string, "ClassPath"=w812:path)  [unwired: 9 in, 8 out]
                          n380 = Empty String/Path?(string/path=w812) -> (empty?=w817:bool)
                          n381 = Concatenate Strings(w818, ".llb" ("string")) -> (w825:string)
                          n382 = Empty String/Path?(string/path=w809) -> (empty?=w810:bool)
                          n383 = call <resource>:"UMLEditor_RelativePath.vi"("Path In"=w809) -> ("ConvertToAbsolutePath(If possible)"=w808:path)  [unwired: 1 in, 17 out]
                          n384 = Select(t=w809, s=w810, f=w808) -> (s? t:f=w807:path)
                          n385 = Select(t=w807, s=w817, f=w812) -> (s? t:f=w816:path)
                          n386 = call <resource>:"Common_DoesClassExist.vi"("ClassPath"=w816, "ClassName"=w818) -> ("ClassExists"=w823:bool, "llb-class"=w822:bool, "llb/LvCLass-Path"=w821:path)  [unwired: 15 out]
                          n387 = case shown="True" w823 {
                            tunnel: [w831 w836] -> w826
                            tunnel: w825 -> [w830 _]
                            tunnel: w824 -> [w829 _]
                            tunnel: w816 -> [w828 w837]
                            tunnel: w822 -> [_ w839]
                            tunnel: w821 -> [_ w838]
                            frame False {
                              n388 = case shown="False" w829 {
                                tunnel: w828 -> [w834 w835]
                                tunnel: [w833 w835] -> w831
                                tunnel: w830 -> [w832 _]
                                frame False {
                                n389 = Build Path(base path=w834, name or relative path=w832) -> (appended path=w833:path)
                                }
                                frame True {
                                }
                              }
                            }
                            frame True {
                              n390 = Select(t=w838, s=w839, f=w837) -> (s? t:f=w836:path)
                            }
                          }
                        }
                        frame Disabled {
                          n391 = Index Array(array=w851, index=w847) -> (element=w850:T15)
                          n392 = Unbundle By Name(w850) -> ("Class folder"=w842:path, "ClassName"=w844:string)
                          n393 = Concatenate Strings(w844, ".llb" ("string")) -> (w846:string)
                          n394 = call <resource>:"Common_DoesClassExist.vi"("ClassPath"=w842, "ClassName"=w844) -> ("ClassExists"=w843:bool, "llb-class"=w841:bool, "llb/LvCLass-Path"=w840:path)  [unwired: 15 out]
                          n395 = case shown="True" w843 {
                            tunnel: [w855 w860] -> w848
                            tunnel: w846 -> [w854 _]
                            tunnel: w845 -> [w853 _]
                            tunnel: w842 -> [w852 w861]
                            tunnel: w841 -> [_ w863]
                            tunnel: w840 -> [_ w862]
                            frame False {
                              n396 = case shown="True" w853 {
                                tunnel: w852 -> [w858 w859]
                                tunnel: [w857 w859] -> w855
                                tunnel: w854 -> [w856 _]
                                frame False {
                                n397 = Build Path(base path=w858, name or relative path=w856) -> (appended path=w857:path)
                                }
                                frame True {
                                }
                              }
                            }
                            frame True {
                              n398 = Select(t=w862, s=w863, f=w861) -> (s? t:f=w860:path)
                            }
                          }
                        }
                        frame Disabled {
                          n399 = Index Array(array=w872, index=w871) -> (element=w865:refnum<class "ClassNode.lvclass">)
                          n400 = call-dynamic "getClassInfo.vi"("reference"=w865) -> ("className"=w870:string, "ClassPath"=w867:path)  [unwired: 9 in, 8 out]
                          n401 = call <resource>:"Common_DoesClassExist.vi"("ClassPath"=w867, "ClassName"=w870) -> ("ClassExists"=w869:bool, "llb-class"=w868:bool, "llb/LvCLass-Path"=w866:path)  [unwired: 15 out]
                          n402 = case shown="False" w869 {
                            tunnel: w868 -> [_ w877]
                            tunnel: [_ w876] -> w864
                            tunnel: w867 -> [_ w875]
                            tunnel: w866 -> [_ w874]
                            frame False {
                              n403 = One Button Dialog(message="Warning\nThis class inherits an other class.\nBut this base class can't be found.\nThis could be because the base class has\nno Class Path Defined, or this base class\nhas not been created yet.") -> ()  [unwired: 2 out]
                            }
                            frame True {
                              n404 = case shown="False" w877 {
                                tunnel: [w878 w879] -> w876
                                tunnel: w875 -> [w878 _]
                                tunnel: w874 -> [_ w879]
                                frame False {
                                }
                                frame True {
                                }
                              }
                            }
                          }
                        }
                      }
                    }
                    frame True {
                      n405 = call-dynamic "getClassInfo.vi"("reference"=w886) -> ("className"=w885:string, "ClassPath"=w881:path)  [unwired: 9 in, 8 out]
                      n406 = call <resource>:"Common_DoesClassExist.vi"("ClassPath"=w881, "ClassName"=w885) -> ("ClassExists"=w884:bool, "llb-class"=w883:bool, "llb/LvCLass-Path"=w880:path)  [unwired: 15 out]
                      n407 = case shown="True" w884 {
                        tunnel: w883 -> [_ w890]
                        tunnel: [_ w889] -> w882
                        tunnel: w881 -> [_ w888]
                        tunnel: w880 -> [_ w887]
                        frame False {
                        }
                        frame True {
                          n408 = case shown="False" w890 {
                            tunnel: [w891 w892] -> w889
                            tunnel: w888 -> [w891 _]
                            tunnel: w887 -> [_ w892]
                            frame False {
                            }
                            frame True {
                            }
                          }
                        }
                      }
                    }
                  }
                  n409 = Index Array(array=w796, index=w788) -> (element=w799:T15)
                  n410 = Bundle By Name(cluster=w799, "ClassType"=w791, "Base class"=w787) -> (w798:T15)
                  n411 = Replace Array Subset(array=w796, new element=w798, index=w788) -> (w797:T15[])
                  n412 = Empty String/Path?(string/path=w787) -> (empty?=w786:bool)
                }
              }
            }
            "classes" <- w748
            n413 = Bundle By Name(cluster=w754, "classes"=w748) -> (w753:T16)
            n414 = case shown="True" w741 {
              frame False {
              }
              frame True {
                n415 = One Button Dialog(message="Warning\nThis class inherits an other class.\nBut this base class can't be found.\nThis could be because the base class has\nno Class Path Defined, or this base class\nhas not been created yet.", button name ("OK")="Abort") -> ()  [unwired: 1 out]
              }
            }
            n416 = Select(t="Exit" ("y"), s=w741, f="CheckIfClassExistsInProject" ("y")) -> (s? t:f=w742:string)
          }
          frame "CheckIfClassExistsInProject" {
            w897 = TRUE ("ExcludeDependencies")
            n417 = call <resource>:"CommonVIs_UmlOpenVIRef.vi"("error in"=w913) -> ("error out"=w914:errorcluster, "ProjectNameOut"=w896:string, "AppRefOut"=w895:refnum<vi>)  [unwired: 3 in, 5 out]
            n418 = Unbundle By Name(w901) -> ("classes"=w915:T15[])
            n419 = property class="App"(reference=w895) -> (error out=w894:errorcluster, "Project.TargetItem"=w893:refnum<vi>)  [unwired: 1 in, 1 out]
            n420 = case shown="No Error" w894 {
              tunnel: w914 -> [w916 w926]
              tunnel: [w916 w923] -> w912
              tunnel: [w917 w918] -> w906
              tunnel: [_ w922] -> w903
              tunnel: w896 -> [_ w921]
              tunnel: w893 -> [w917 _]
              frame No Error {
              }
              frame Error {
                n421 = call <resource>:"GDSProject_GetProjects.vi"("GetProjectRefByName"=w921, "error in (no error)"=w926) -> ("Project Refnum"=w925:refnum<vi>, "error out"=w924:errorcluster)  [unwired: 1 in, 15 out]
                n422 = property class="Project"(reference=w925, error in=w924) -> (reference out=w922:refnum<vi>, error out=w923:errorcluster, "My Computer"=w919:refnum<vi>)
                n423 = To More Generic Class(target class=refnum<vi> refnum ("My Computer"), reference=w919) -> (generic class reference=w918:refnum<vi>)
              }
            }
            n424 = invoke class="ProjectItem" method="Get All Descendents"(reference=w906, error in=w912, "Type"="lvclass", "Exclude Dependencies"=w897, "ExcludeBuilds"=w897) -> (reference out=w907:refnum<vi>, error out=w909:errorcluster, "All Descendents"=w910:refnum<vi>[])  [unwired: 2 in, 4 out]
            n425 = for {
              tunnel: w910 -> [w933] mode=indexing
              shift-right: [w928] -> w905
              shift-left: w909 -> [w932]
              tunnel: [w931] -> w908 mode=indexing
              tunnel: [w930] -> w898 mode=indexing
              n426 = property class="ProjectItem"(reference=w933, error in=w932) -> (reference out=w929:refnum<vi>, error out=w927:errorcluster, "Path"=w930:path)
              n427 = Strip Path(path=w930) -> (stripped path=w931:path)  [unwired: 1 out]
              n428 = Close Reference(reference=w929, error in (no error)=w927) -> (error out=w928:errorcluster)
            }
            n429 = for {
              tunnel: w915 -> [w945] mode=indexing
              tunnel: w908 -> [w943]
              tunnel: [w940] -> w900 mode=indexing
              tunnel: w898 -> [w938]
              n430 = Unbundle By Name(w945) -> ("ExistsAsFile"=w944:bool, "Class folder"=w937:path)
              n431 = Search 1D Array(1D array=w943, element=w937) -> (index of element=w941:i32)  [unwired: 1 out]
              n432 = Search 1D Array(1D array=w938, element=w937) -> (index of element=w939:i32)  [unwired: 1 out]
              n433 = Greater Or Equal To 0?(x=w941) -> (x >= 0?=w935:bool)
              n434 = Greater Or Equal To 0?(x=w939) -> (x >= 0?=w934:bool)
              n435 = Or(x=w935, y=w934) -> (x .or. y?=w936:bool)
              n436 = And(x=w944, y=w936) -> (x .and. y?=w942:bool)
              n437 = Bundle By Name(cluster=w945, "ExistsInProject"=w942) -> (w940:T15)
            }
            n438 = Bundle By Name(cluster=w901, "classes"=w900) -> (w899:T16)
            n439 = Close Reference(reference=w907, error in (no error)=w905) -> (error out=w904:errorcluster)
            n440 = Close Reference(reference=w903, error in (no error)=w904) -> ()  [unwired: 1 out]
          }
          frame "CheckForClassTemplateToUse(Stereotype)" {
            # "If stereotype used, try to find a template class to use as ClassTemplateOption"
            n441 = Unbundle By Name(w957) -> ("ClassWriterRef"=w951:refnum<class "ClassWriter.lvclass">, "classes"=w952:T15[])
            n442 = for {
              shift-right: [w964] -> w953
              shift-left: w954 -> [w966]
              tunnel: w952 -> [w967] mode=indexing
              tunnel: [w968] -> w950 mode=indexing
              tunnel: w951 -> [w963]
              n443 = Unbundle By Name(w967) -> ("ClassType"=w961:i32, "BaseClass"=w958:bool, "ClassStereotype"=w959:string)
              n444 = case shown="Default" w959 {
                selector: w959 -> [w974 _]
                tunnel: w966 -> [w978 w979]
                tunnel: [w976 w979] -> w965
                tunnel: w963 -> [w977 _]
                tunnel: [w973 _] -> w962
                tunnel: [w972 _] -> w960
                tunnel: w958 -> [w970 _]
                frame Default {
                  n445 = call-dynamic "GetTemplatePath.vi"("ClassWriterIn"=w977, "ClassTemplateSubDirectory"=w974, "error in (no error)"=w978) -> ("FolderPathOut"=w975:path, "error out"=w976:errorcluster)  [unwired: 15 out]
                  n446 = local read "Connector Pane Pattern"() -> (w971:T1)
                  n447 = Not(x=w970) -> (.not. x?=w969:bool)
                  n448 = call <resource>:"UMLEditor_GetStereoTypeTemplate.vi"("SubClass"=w969, "Connector Pane Pattern"=w971, "String in"=w974, "FolderPathOut"=w975) -> ("FoundTemplate"=w973:bool, "TemplateToUse"=w972:string)  [unwired: 6 in]
                }
                frame "" {
                }
              }
              n449 = case shown="False" w962 {
                tunnel: w967 -> [w991 w1001]
                tunnel: [w990 w1000] -> w968
                tunnel: w959 -> [_ _]
                tunnel: w965 -> [w994 w999]
                tunnel: [w993 w999] -> w964
                tunnel: w963 -> [w992 _]
                tunnel: w961 -> [w985 _]
                tunnel: w960 -> [_ w998]
                frame False {
                  w984 = 1 items=["Standard class", "Sub class from an existing base class", "Clone class from an existing class"] ("ClassType")
                  n450 = call-dynamic "GetClassTemplates.vi"("ClassWriter in"=w992, "error in (no error)"=w994) -> ("Templates"=w989:T45[], "error out"=w993:errorcluster)  [unwired: 1 in, 15 out]
                  n451 = for {
                    tunnel: w989 -> [w997] mode=indexing
                    tunnel: [w996] -> w988 mode=indexing
                    tunnel: [w995] -> w987 mode=indexing
                    n452 = Unbundle By Name(w997) -> ("TemplateIdName"=w995:string, "OnlySubClassTemplate"=w996:bool)  [unwired: 1 out]
                  }
                  n453 = Equal?(x=w985, y=w984) -> (x = y?=w983:bool)
                  n454 = Search 1D Array(1D array=w988, element=w983) -> (index of element=w982:i32)  [unwired: 1 out]
                  n455 = Max & Min(x=w982, y=0) -> (max(x,y)=w981:i32)  [unwired: 1 out]
                  n456 = Index Array(array=w987, index=w981) -> (element=w986:string)
                  n457 = Bundle By Name(cluster=w991, "ClassTemplateOption"=w986) -> (w990:T15)
                }
                frame True {
                  n458 = Bundle By Name(cluster=w1001, "ClassTemplateOption"=w998) -> (w1000:T15)
                }
              }
            }
            n459 = Array Size(array=w950) -> (size(s)=w947:i32)
            n460 = Format Into String(format string="Creating %d classes", w947) -> (resulting string=w946:string)  [unwired: 2 in, 1 out]
            n461 = control-ref of="Class creation progress"() -> (w949:refnum<vi>)
            n462 = call <resource>:"UMLEditor createWizardScriptFile_UpdateList.vi"("String"=w946, "Progress"=w949) -> ()  [unwired: 9 in, 1 out]
            n463 = Bundle By Name(cluster=w957, "classes"=w950) -> (w956:T16)
          }
          frame "UpdateAfStereoTypeWithNoBaseClass" {
            # "If stereotype used, try to find a template class to use as ClassTemplateOption"
            n464 = Unbundle By Name(w1013) -> ("ClassWriterRef"=w1008:refnum<class "ClassWriter.lvclass">, "classes"=w1009:T15[])
            n465 = for {
              shift-right: [w1023] -> w1010
              shift-left: w1011 -> [w1021]
              tunnel: w1009 -> [w1024] mode=indexing
              tunnel: [w1025] -> w1007 mode=indexing
              tunnel: w1008 -> [w1022]
              n466 = Unbundle By Name(w1024) -> ("Class folder"=w1019:path, "ClassStereotype"=w1020:string)
              n467 = To Upper Case(1:w1020) -> (0:w1017:string)
              n468 = Equal?(x=w1017, y="ACTOR") -> (x = y?=w1016:bool)
              n469 = Empty String/Path?(string/path=w1019) -> (empty?=w1015:bool)
              n470 = Compound Arithmetic op=AND(w1015, w1016) -> (w1014:bool)
              n471 = case shown="True" w1014 {
                tunnel: w1024 -> [w1054 w1062]
                tunnel: [w1053 w1062] -> w1025
                tunnel: w1021 -> [w1052 w1063]
                tunnel: [w1027 w1063] -> w1023
                tunnel: w1022 -> [_ _]
                frame True {
                  n472 = call <resource>:"CommonVIs_UmlOpenVIRef.vi"("error in"=w1052) -> ("error out"=w1041:errorcluster, "AppRefOut"=w1051:refnum<vi>)  [unwired: 3 in, 6 out]
                  n473 = property class="App"(reference=w1051, error in=w1041) -> (error out=w1044:errorcluster, "Project.TargetItem"=w1026:refnum<vi>)  [unwired: 1 out]
                  n474 = invoke class="TargetItem" method="Get All Descendents"(reference=w1026, error in=w1044, "Type"="Library") -> (error out=w1043:errorcluster, "All Descendents"=w1049:refnum<vi>[])  [unwired: 4 in, 5 out]
                  n475 = VI Library() -> (path=w1037:path)
                  n476 = Strip Path(path=w1037) -> (stripped path=w1038:path)  [unwired: 1 out]
                  n477 = for {
                    tunnel: w1049 -> [w1061] mode=indexing
                    tunnel: [w1059] -> w1047
                    tunnel: [w1057] -> w1046
                    shift-right: [w1055] -> w1042
                    shift-left: w1043 -> [w1056]
                    stop <- w1059 stop-if-true
                    n478 = property class="ProjectItem"(reference=w1061, error in=w1056) -> (error out=w1055:errorcluster, "Name"=w1058:string, "Path"=w1057:path)  [unwired: 1 out]
                    n479 = Equal?(x=w1058, y="Actor Framework.lvlib") -> (x = y?=w1059:bool)
                  }
                  n480 = Build Path(base path=w1037, name or relative path=path "ActorFramework/Actor Framework.lvlib" ("stripped path")) -> (appended path=w1040:path)
                  n481 = Build Path(base path=w1038, name or relative path=path "user.lib/_Frameworks/Actor Framework/Actor Framework.lvlib" ("stripped path")) -> (appended path=w1031:path)
                  n482 = call <vilib>:"Check if File or Folder Exists.vi"("path"=w1031) -> ("file or folder exists?"=w1032:bool, "dup path"=w1033:path)  [unwired: 8 in, 1 out]
                  n483 = call <vilib>:"Check if File or Folder Exists.vi"("path"=w1040) -> ("file or folder exists?"=w1036:bool, "dup path"=w1035:path)  [unwired: 8 in, 1 out]
                  n484 = Select(t=w1033, s=w1032, f=path "") -> (s? t:f=w1030:path)
                  n485 = Select(t=w1035, s=w1036, f=w1030) -> (s? t:f=w1034:path)
                  n486 = Close Reference(reference=w1049, error in (no error)=w1042) -> (error out=w1028:errorcluster)
                  n487 = Select(t=w1046, s=w1047, f=w1034) -> (s? t:f=w1045:path)
                  n488 = Bundle By Name(cluster=w1054, "Base class"=w1045) -> (w1053:T15)
                  n489 = Close Reference(reference=w1026, error in (no error)=w1028) -> (error out=w1027:errorcluster)
                }
                frame False {
                }
              }
            }
            n490 = Array Size(array=w1007) -> (size(s)=w1004:i32)
            n491 = Format Into String(format string="Creating %d classes", w1004) -> (resulting string=w1003:string)  [unwired: 2 in, 1 out]
            n492 = control-ref of="Class creation progress"() -> (w1006:refnum<vi>)
            n493 = call <resource>:"UMLEditor createWizardScriptFile_UpdateList.vi"("String"=w1003, "Progress"=w1006) -> ()  [unwired: 9 in, 1 out]
            n494 = Bundle By Name(cluster=w1013, "classes"=w1007) -> (w1012:T16)
          }
          frame "UpdateAfClassTemplate" {
            # "If stereotype used, try to find a template class to use as ClassTemplateOption"
            n495 = Unbundle By Name(w1076) -> ("G4"=w1065:bool, "ClassWriterRef"=w1071:refnum<class "ClassWriter.lvclass">, "classes"=w1072:T15[])
            n496 = for {
              shift-right: [w1087] -> w1073
              shift-left: w1074 -> [w1083]
              tunnel: w1072 -> [w1088] mode=indexing
              tunnel: [w1089] -> w1070 mode=indexing
              tunnel: w1071 -> [w1086]
              tunnel: w1065 -> [w1084]
              n497 = Unbundle By Name(w1088) -> ("ClassTemplateOption"=w1085:string, "Class folder"=w1077:path, "Base class"=w1078:path)
              n498 = call <vilib>:"Check if File or Folder Exists.vi"("error in (no error)"=w1083, "path"=w1078) -> ("error out"=w1079:errorcluster, "file or folder exists?"=w1082:bool)  [unwired: 7 in, 1 out]
              n499 = Empty String/Path?(string/path=w1078) -> (empty?=w1081:bool)
              n500 = Compound Arithmetic op=AND(invert w1081, w1082) -> (w1080:bool)
              n501 = case shown="True" w1080 {
                tunnel: w1088 -> [w1091 w1094]
                tunnel: [w1091 w1093] -> w1089
                tunnel: w1085 -> [_ w1103]
                tunnel: w1079 -> [w1090 w1099]
                tunnel: [w1090 w1097] -> w1087
                tunnel: w1086 -> [_ _]
                tunnel: w1084 -> [_ w1102]
                tunnel: w1078 -> [_ w1098]
                tunnel: w1077 -> [_ w1092]
                frame False {
                }
                frame True {
                  n502 = call <resource>:"CommonVIs_UmlOpenVIRef.vi"("error in"=w1099) -> ("error out"=w1100:errorcluster, "AppRefOut"=w1101:refnum<vi>)  [unwired: 3 in, 6 out]
                  n503 = invoke class="App" method="LVClass.Open"(reference=w1101, error in=w1100, "Path"=w1098) -> (error out=w1097:errorcluster, "LVClass.Open"=w1096:refnum<vi>)  [unwired: 1 in, 2 out]
                  n504 = call <resource>:"AF_GetClassAfInfo.vi"("DeriveFromClassRef"=w1096) -> ("TemplateIdName"=w1105:string, "RootClassQualifiedName"=w1104:string)  [unwired: 5 in, 4 out]
                  n505 = case shown="Default" w1104 {
                    tunnel: w1105 -> [_ w1122]
                    tunnel: w1103 -> [w1106 w1123]
                    tunnel: w1102 -> [_ w1121]
                    tunnel: [w1109 w1120] -> w1095
                    tunnel: w1096 -> [w1109 w1120]
                    tunnel: w1094 -> [w1108 w1118]
                    tunnel: [w1107 w1117] -> w1093
                    tunnel: w1092 -> [_ w1114]
                    frame Default {
                      n506 = Bundle By Name(cluster=w1108, "ClassTemplateOption"=w1106) -> (w1107:T15)
                    }
                    frame "Actor Framework.lvlib:Actor.lvclass" {
                      n507 = Strip Path(path=w1114) -> (stripped path=w1113:path)  [unwired: 1 out]
                      n508 = case shown="\"4.0.0\", Default" w1122 {
                        tunnel: [w1127 w1131] -> w1124
                        tunnel: w1121 -> [w1126 w1130]
                        frame "3.0.7" {
                          n509 = case shown="True" w1126 {
                            tunnel: ["Actor1_Basic_G4_3.0.7" ("format string") "Actor1_Basic_N_3.0.7" ("format string")] -> w1127
                            frame True {
                            }
                            frame False {
                            }
                          }
                        }
                        frame "4.0.0", Default {
                          n510 = case shown="False" w1130 {
                            tunnel: ["Actor1_Basic_G4_4.0.0" ("format string") "Actor1_Basic_N_4.0.0" ("format string")] -> w1131
                            frame True {
                            }
                            frame False {
                            }
                          }
                        }
                      }
                      n511 = Strip Path(path=w1113) -> (stripped path=w1112:path, name=w1116:string)
                      n512 = Match Pattern(string=w1116, regular expression="_class") -> (before substring=w1111:string)  [unwired: 1 in, 3 out]
                      n513 = Build Path(base path=w1112, name or relative path=w1111) -> (appended path=w1110:path)
                      n514 = Format Into String(format string="AF%s_%s+%s", w1122, w1124, w1123) -> (resulting string=w1119:string)  [unwired: 2 in, 1 out]
                      n515 = Bundle By Name(cluster=w1118, "ClassTemplateOption"=w1119, "Class folder"=w1110) -> (w1117:T15)
                    }
                  }
                  n516 = Close Reference(reference=w1095, error in (no error)=w1097) -> ()  [unwired: 1 out]
                }
              }
            }
            n517 = Array Size(array=w1070) -> (size(s)=w1067:i32)
            n518 = Format Into String(format string="Creating %d classes", w1067) -> (resulting string=w1066:string)  [unwired: 2 in, 1 out]
            n519 = control-ref of="Class creation progress"() -> (w1069:refnum<vi>)
            n520 = call <resource>:"UMLEditor createWizardScriptFile_UpdateList.vi"("String"=w1066, "Progress"=w1069) -> ()  [unwired: 9 in, 1 out]
            n521 = Bundle By Name(cluster=w1076, "classes"=w1070) -> (w1075:T16)
          }
          frame "GetParentInterfaces" {
            n522 = Unbundle By Name(w1136) -> ("classes"=w1143:T15[], "InterfaceEdges"=w1140:refnum<class "ClassRelationshipEdge.lvclass">[])
            n523 = Unbundle By Name(w1136) -> ("classes"=w1134:T15[])
            n524 = for {
              tunnel: w1134 -> [w1146] mode=indexing
              tunnel: [w1145] -> w1135 mode=indexing
              n525 = Unbundle By Name(w1146) -> ("Node"=w1145:refnum<class "ClassNode.lvclass">)
            }
            n526 = for {
              tunnel: w1140 -> [w1149] mode=indexing
              tunnel: [w1148] -> w1139 mode=indexing
              tunnel: [w1147] -> w1138 mode=indexing
              n527 = call <resource>:"WhoInheritsWhom.vi"("reference"=w1149) -> ("inherits"=w1148:refnum<class "AbstractNode.lvclass">, "base"=w1147:refnum<class "AbstractNode.lvclass">)  [unwired: 1 in, 16 out]
            }
            n528 = for {
              tunnel: w1143 -> [w1157] mode=indexing
              tunnel: [w1158] -> w1141 mode=indexing
              tunnel: w1139 -> [w1156]
              tunnel: w1138 -> [w1154]
              tunnel: w1135 -> [w1152]
              tunnel: w1134 -> [w1151]
              n529 = Unbundle By Name(w1157) -> ("Node"=w1155:refnum<class "ClassNode.lvclass">)
              n530 = while {
                tunnel: w1156 -> [w1170]
                tunnel: w1155 -> [w1169]
                tunnel: w1154 -> [w1167]
                shift-right: [w1165] -> _
                shift-left: 0 -> [w1166]
                tunnel: w1152 -> [w1163]
                tunnel: w1151 -> [w1162]
                tunnel: [w1161] -> w1150 mode=indexing if=w1159
                stop <- w1164 stop-if-true
                n531 = Search 1D Array(1D array=w1170, element=w1169, start index (0)=w1166) -> (index of element=w1168:i32)
                n532 = case shown="0, Default" w1168 {
                  selector: w1168 -> [w1183 _]
                  tunnel: w1167 -> [w1191 _]
                  tunnel: [w1189 _] -> w1165
                  tunnel: [_ TRUE] -> w1164
                  tunnel: w1163 -> [w1188 _]
                  tunnel: w1162 -> [w1185 _]
                  tunnel: [w1171 _] -> w1161
                  frame 0, Default {
                    n533 = Index Array(array=w1191, index=w1183) -> (element=w1187:refnum<class "AbstractNode.lvclass">)
                    n534 = To More Specific Class(target class=refnum<class "ClassNode.lvclass"> refnum ("reference"), reference=w1187) -> (specific class reference=w1186:refnum<class "ClassNode.lvclass">)  [unwired: 1 in, 1 out]
                    n535 = Search 1D Array(1D array=w1188, element=w1186) -> (index of element=w1184:i32)  [unwired: 1 in]
                    n536 = Index Array(array=w1185, index=w1184) -> (element=w1172:T15)
                    n537 = Increment(x=w1183) -> (x+1=w1189:i32)
                    n538 = Unbundle By Name(w1172) -> ("ClassName"=w1178:string, "Class folder"=w1175:path)
                    n539 = call <vilib>:"Get File Extension.vi"("file"=w1175) -> ("lowercase file extension"=w1179:string, "dup file"=w1182:path)  [unwired: 1 in, 8 out]
                    n540 = Strip Path(path=w1175) -> (stripped path=w1181:path)  [unwired: 1 out]
                    n541 = Not Equal?(x=w1179, y="lvclass") -> (x != y?=w1180:bool)
                    n542 = Concatenate Strings(w1178, ".lvclass" ("string")) -> (w1176:string)
                    n543 = Select(t=w1182, s=w1180, f=w1181) -> (s? t:f=w1177:path)
                    n544 = Build Path(base path=w1177, name or relative path=w1176) -> (appended path=w1171:path)
                  }
                  frame -1 {
                  }
                }
                n545 = Empty String/Path?(string/path=w1161) -> (empty?=w1160:bool)
                n546 = Not(x=w1160) -> (.not. x?=w1159:bool)
              }
              n547 = Bundle By Name(cluster=w1157, "ParentInterfaces"=w1150) -> (w1158:T15)
            }
            n548 = Bundle By Name(cluster=w1136, "classes"=w1141) -> (w1142:T16)
          }
          frame "ArrangeCreationOrder" {
            # "Use a for loop with a fixed number of Max iterations, if we get a circular dependency we want to stop after a while.\nGo though all classes, if this class has a base class or a parent interfaec class that havn't been created yet move it to the end."
            n549 = Unbundle By Name(w1197) -> ("classes"=w1202:T15[], "InterfaceEdges"=w1200:refnum<class "ClassRelationshipEdge.lvclass">[])
            n550 = for {
              tunnel: w1200 -> [w1206] mode=indexing
              tunnel: [w1205] -> w1199 mode=indexing
              tunnel: [w1204] -> w1198 mode=indexing
              n551 = call <resource>:"WhoInheritsWhom.vi"("reference"=w1206) -> ("inherits"=w1205:refnum<class "AbstractNode.lvclass">, "base"=w1204:refnum<class "AbstractNode.lvclass">)  [unwired: 1 in, 16 out]
            }
            n552 = for {
              N: 1000 -> [_]
              tunnel: w1199 -> [_]
              tunnel: w1198 -> [_]
              shift-right: [w1209] -> _
              shift-left: w1202 -> [w1236]
              tunnel: [w1233] -> w1193 mode=indexing if=w1210
              shift-right: [w1222] -> _
              shift-left: path[] [] -> [w1221]
              stop <- w1208 stop-if-true
              n553 = Delete From Array(array=w1236, index=0) -> (deleted portion=w1233:T15, array with subset deleted=w1234:T15[])  [unwired: 1 in]
              n554 = Unbundle By Name(w1233) -> ("Base class"=w1219:path, "ParentInterfaces"=w1220:path[])
              n555 = for {
                tunnel: w1221 -> [w1240]
                tunnel: w1220 -> [w1239] mode=indexing
                tunnel: [w1237] -> w1217 mode=indexing
                n556 = Search 1D Array(1D array=w1240, element=w1239) -> (index of element=w1238:i32)  [unwired: 1 in]
                n557 = Greater Or Equal To 0?(x=w1238) -> (x >= 0?=w1237:bool)
              }
              n558 = Empty Array?(array=w1220) -> (empty?=w1213:bool)
              n559 = Empty String/Path?(string/path=w1219) -> (empty?=w1215:bool)
              n560 = Search 1D Array(1D array=w1221, element=w1219) -> (index of element=w1218:i32)  [unwired: 1 in]
              n561 = And Array Elements(Boolean array=w1217) -> (logical AND=w1214:bool)
              n562 = Greater Or Equal To 0?(x=w1218) -> (x >= 0?=w1216:bool)
              n563 = Compound Arithmetic op=OR(w1213, w1214) -> (w1211:bool)
              n564 = Unbundle By Name(w1233) -> ("ClassName"=w1227:string, "Class folder"=w1207:path)
              n565 = Compound Arithmetic op=OR(w1215, w1216) -> (w1212:bool)
              n566 = call <vilib>:"Get File Extension.vi"("file"=w1207) -> ("lowercase file extension"=w1229:string, "dup file"=w1232:path)  [unwired: 1 in, 8 out]
              n567 = Compound Arithmetic op=AND(w1212, w1211) -> (w1210:bool)
              n568 = Strip Path(path=w1207) -> (stripped path=w1231:path)  [unwired: 1 out]
              n569 = Not Equal?(x=w1229, y="lvclass") -> (x != y?=w1230:bool)
              n570 = Concatenate Strings(w1227, ".lvclass" ("string")) -> (w1224:string)
              n571 = Select(t=w1232, s=w1230, f=w1231) -> (s? t:f=w1225:path)
              n572 = Build Path(base path=w1225, name or relative path=w1224) -> (appended path=w1223:path)
              n573 = case shown="True" w1210 {
                tunnel: w1234 -> [w1247 w1248]
                tunnel: [w1246 w1248] -> w1209
                tunnel: w1233 -> [w1245 _]
                frame False {
                  n574 = Build Array (concatenate)(w1247, w1245) -> (w1246:T15[])
                }
                frame True {
                }
              }
              n575 = case shown="True" w1210 {
                tunnel: w1221 -> [w1241 w1244]
                tunnel: w1223 -> [_ w1243]
                tunnel: [w1241 w1242] -> w1222
                frame False {
                }
                frame True {
                  n576 = Build Array (concatenate)(w1244, w1243) -> (w1242:path[])
                }
              }
              n577 = Empty Array?(array=w1209) -> (empty?=w1208:bool)
            }
            n578 = Bundle By Name(cluster=w1197, "classes"=w1193) -> (w1201:T16)
          }
          frame "CreateClasses" {
            # "If class don't exists Use Default Provider\nElse Check if class exists in project, if not add it."
            n579 = Unbundle By Name(w1250) -> ("My Computer"=w1257:refnum<vi>, "ClassWriterRef"=w1256:refnum<class "ClassWriter.lvclass">, "classes"=w1255:T15[])
            n580 = while {
              shift-right: [w1282] -> _
              shift-left: w1255 -> [w1291]
              shift-right: [w1277] -> w1253
              shift-left: w1258 -> [w1289]
              tunnel: w1256 -> [w1288]
              tunnel: w1257 -> [w1287]
              shift-right: [w1267] -> w1251
              shift-left: T15[] [] -> [w1269]
              tunnel: w1249 -> [w1263]
              i -> [w1281]
              stop <- w1279 stop-if-true
              n581 = Delete From Array(array=w1291, index=0) -> (deleted portion=w1262:T15, array with subset deleted=w1284:T15[])  [unwired: 1 in]
              n582 = Unbundle By Name(w1262) -> ("Interface"=w1260:bool, "ParentInterfaces"=w1261:path[])
              n583 = Unbundle By Name(w1262) -> ("ExistsAsFile"=w1290:bool, "ExistsInProject"=w1272:bool, "ClassName"=w1271:string, "Class folder"=w1274:path, "Base class"=w1286:path, "ClassIconInfo"=w1285:T46, "ClassTemplateOption"=w1273:string, "ClassStereotype"=w1266:string, "Class description"=w1265:string)  [unwired: 3 out]
              n584 = case shown="False" w1260 {
                tunnel: w1266 -> [w1294 _]
                tunnel: w1265 -> [w1293 w1300]
                tunnel: [w1292 w1300] -> w1264
                frame False {
                  n585 = case shown="Default" w1294 {
                    selector: w1294 -> [_ w1296]
                    tunnel: w1293 -> [w1295 w1298]
                    tunnel: [w1295 w1297] -> w1292
                    frame "" {
                    }
                    frame Default {
                      n586 = Format Into String(format string="<<%s>>\n%s", w1296, w1298) -> (resulting string=w1297:string)  [unwired: 2 in, 1 out]
                    }
                  }
                }
                frame True {
                }
              }
              n587 = case shown="False" w1290 {
                tunnel: w1289 -> [w1318 w1450]
                tunnel: w1288 -> [w1320 _]
                tunnel: w1287 -> [w1319 w1452]
                tunnel: [w1317 w1443] -> w1277
                tunnel: w1286 -> [w1306 _]
                tunnel: w1285 -> [w1315 _]
                tunnel: w1262 -> [w1313 w1447]
                tunnel: [w1312 _] -> w1283
                tunnel: w1271 -> [w1311 w1448]
                tunnel: w1274 -> [w1310 w1451]
                tunnel: w1273 -> [w1309 _]
                tunnel: w1272 -> [_ w1454]
                tunnel: w1271 -> [w1304 _]
                tunnel: [w1308 w1449] -> w1268
                tunnel: w1264 -> [w1307 _]
                tunnel: w1263 -> [_ w1442]
                tunnel: w1260 -> [w1303 _]
                tunnel: w1261 -> [w1302 _]
                frame False {
                  n588 = Empty String/Path?(string/path=w1306) -> (empty?=w1316:bool)
                  n589 = call <vilib>:"Check if File or Folder Exists.vi"("path"=w1306) -> ("file or folder exists?"=w1305:bool)  [unwired: 1 in, 9 out]
                  n590 = call <vilib>:"Trim Whitespace.vi"("string"=w1307) -> ("trimmed string"=w1301:string)  [unwired: 1 in]
                  n591 = Compound Arithmetic op=OR(w1316, w1305) -> (w1314:bool)
                  n592 = case shown="True" w1314 {
                    tunnel: w1320 -> [_ w1338]
                    tunnel: w1319 -> [_ w1330]
                    tunnel: w1318 -> [w1321 w1328]
                    tunnel: [w1321 w1329] -> w1317
                    tunnel: w1315 -> [_ w1337]
                    tunnel: w1313 -> [w1323 w1332]
                    tunnel: [w1322 _] -> w1312
                    tunnel: w1311 -> [_ w1327]
                    tunnel: w1310 -> [_ w1333]
                    tunnel: w1301 -> [_ w1336]
                    tunnel: w1309 -> [_ w1335]
                    tunnel: w1306 -> [_ w1334]
                    tunnel: [_ w1331] -> w1308
                    tunnel: w1304 -> [_ w1326]
                    tunnel: w1303 -> [_ w1325]
                    tunnel: w1302 -> [_ w1324]
                    frame False {
                      n593 = Build Array(w1323) -> (w1322:T15[])
                    }
                    frame True {
                      n594 = case shown="True" w1325 {
                        tunnel: w1338 -> [w1343 w1437]
                        tunnel: w1337 -> [w1386 w1412]
                        tunnel: w1336 -> [w1370 w1401]
                        tunnel: w1335 -> [w1369 _]
                        tunnel: w1334 -> [w1368 _]
                        tunnel: w1333 -> [w1364 w1403]
                        tunnel: w1332 -> [w1362 w1439]
                        tunnel: [w1360 w1438] -> w1331
                        tunnel: w1330 -> [w1358 w1411]
                        tunnel: [w1342 w1397] -> w1329
                        tunnel: w1328 -> [w1355 w1416]
                        tunnel: w1327 -> [w1354 w1408]
                        tunnel: w1326 -> [w1347 w1415]
                        tunnel: w1324 -> [w1344 w1399]
                        tunnel: [w1339 w1395] -> _
                        frame False {
                          n595 = Unbundle By Name(w1386) -> ("Frame color"=w1378:u32, "Foreground color"=w1373:u32, "Header color"=w1372:u32, "Public color"=w1377:u32, "Protected color"=w1376:u32, "Private color"=w1375:u32, "Icon class name"=w1374:string)
                          n596 = call <vilib>:"Get File Extension.vi"("file"=w1364) -> ("lowercase file extension"=w1367:string, "dup file"=w1356:path)  [unwired: 1 in, 8 out]
                          n597 = call <resource>:"GOOP_DebugLogger.vi"("error in (no error)"=w1355, "Data"=w1354, "State"="## Create Class ##") -> ("error out"=w1352:errorcluster)  [unwired: 6 in, 2 out]
                          n598 = Strip Path(path=w1364) -> (stripped path=w1363:path)  [unwired: 1 out]
                          n599 = Format Into String(format string="Creating Class %s", w1347) -> (resulting string=w1346:string)  [unwired: 2 in, 1 out]
                          n600 = Not Equal?(x=w1367, y="lvclass") -> (x != y?=w1365:bool)
                          n601 = Select(t=w1356, s=w1365, f=w1363) -> (s? t:f=w1357:path)
                          n602 = call <resource>:"UMLEditor createWizardScriptFile_UpdateList.vi"("error in (no error)"=w1352, "String"=w1346) -> ("error out"=w1351:errorcluster)  [unwired: 9 in]
                          n603 = Bundle By Name(cluster=T24 {"ClassName"="", "ClassFolder"=path "", "ClassDescription"="", "ClassTemplateOptions"="", "BaseClass(ProjectStringPath or LvClassFilePath)"=variant, "ExtraCreateParameters"=variant, "FolderSuffix"="", "ParentInterfaces"=[]} ("CreateClassData"), "ClassName"=w1354, "ClassFolder"=w1357, "ClassDescription"=w1370, "ClassTemplateOptions"=w1369, "BaseClass(ProjectStringPath or LvClassFilePath)"=w1368, "FolderSuffix"="_Actor") -> (w1387:T24)
                          n604 = Bundle By Name(cluster=T20 {"Frame"=0, "Header Text Color"=0, "Header Background"=8453954, "BodyBackgroundPublic"=16121600, "BodyBackgroundProtected"=16777215, "BodyBackgroundPrivate"=16777215, "Body Text Color"=1, "Frame thickness"=1, "ProtectedPrivateSame"=FALSE, "Icon Header Size"=7, "Font Compression"=enum."Auto", "CapitalOnly"=TRUE} ("Colors"), "Frame"=w1378, "Header Text Color"=w1373, "Header Background"=w1372, "BodyBackgroundPublic"=w1377, "BodyBackgroundProtected"=w1376, "BodyBackgroundPrivate"=w1375, "Body Text Color"=w1373) -> (w1379:T20)
                          n605 = Bundle(cluster=T21 {"Text"="myhedaer", "Allow Only Capital Chars"=TRUE, "Compression"=enum."Auto", "Alignment"=enum."Center"} ("Text"), "Text"=w1374) -> (w1384:T21)  [unwired: 3 out]
                          n606 = call <resource>:"GDSLvIcon_GenerateIconText.vi"("Text"=w1384, "TextPixelHeight(5-30)"=7, "Foreground color"=w1373, "Background color"=w1372, "error in (no error)"=w1351, "Text Pixel width(32-FrameThicknes*2))"=30) -> ("TextOut"=w1382:u8[][], "error out"=w1350:errorcluster)  [unwired: 2 in, 10 out]
                          n607 = Bundle("Colors"=w1379, "TextOut"=w1382) -> (w1381:cluster{"Colors":T20, "TextOut":u8[][]})  [unwired: 1 out]
                          n608 = call-dynamic "CreateClass.vi"("ClassWriter.lvclass"=w1343, "ProjectTreePosition(String or Project Item Ref)"=w1358, "CreateClassData"=w1387, "error in (no error)"=w1350, "KeepLvClassRefOpen(False)"=TRUE, "HeaderToApply (take from VIRef or /use 2D-8bit header, Ignored if not wired)"=w1381) -> ("LVClassLibraryRefnum"=w1340:refnum<vi>, "error out"=w1345:errorcluster)  [unwired: 1 in, 11 out]
                          n609 = Bundle By Name(cluster=w1362, "LVClassRef"=w1340) -> (w1361:T15)
                          n610 = for {
                            tunnel: w1340 -> [w1392]
                            shift-right: [w1393] -> w1342
                            shift-left: w1345 -> [w1394]
                            tunnel: w1344 -> [w1391] mode=indexing
                            tunnel: w1343 -> [w1389]
                            n611 = call <resource>:"ImplementInterface.vi"("ClassWriter.lvclass"=w1389, "error in"=w1394, "CreateMethods"=FALSE, "Interface Path"=w1391, "LvClassPath/LvClassProjectItem"=w1392) -> ("error out"=w1393:errorcluster)  [unwired: 6 in]
                          }
                          n612 = call <resource>:"GOOP_ApplyOverlayIconFromClassRef.vi"("error in (no error)"=w1342, "LVClassRef"=w1340) -> ("error out"=w1341:errorcluster)  [unwired: 9 in]
                          n613 = Close Reference(reference=w1340, error in (no error)=w1341) -> (error out=w1339:errorcluster)
                          n614 = Build Array(w1361) -> (w1360:T15[])
                        }
                        frame True {
                          n615 = call <vilib>:"Get File Extension.vi"("file"=w1403) -> ("lowercase file extension"=w1407:string, "dup file"=w1400:path)  [unwired: 1 in, 8 out]
                          n616 = Unbundle By Name(w1412) -> ("Frame color"=w1430:u32, "Foreground color"=w1425:u32, "Header color"=w1424:u32, "Public color"=w1429:u32, "Protected color"=w1428:u32, "Private color"=w1427:u32, "Icon class name"=w1426:string)
                          n617 = call <resource>:"GOOP_DebugLogger.vi"("error in (no error)"=w1416, "State"="## Create Interface ##") -> ("error out"=w1421:errorcluster)  [unwired: 7 in, 2 out]
                          n618 = Strip Path(path=w1403) -> (stripped path=w1405:path)  [unwired: 1 out]
                          n619 = Not Equal?(x=w1407, y="lvclass") -> (x != y?=w1406:bool)
                          n620 = Format Into String(format string="Creating Interface %s", w1415) -> (resulting string=w1418:string)  [unwired: 2 in, 1 out]
                          n621 = Select(t=w1400, s=w1406, f=w1405) -> (s? t:f=w1402:path)
                          n622 = call <resource>:"UMLEditor createWizardScriptFile_UpdateList.vi"("error in (no error)"=w1421, "String"=w1418) -> ("error out"=w1420:errorcluster)  [unwired: 9 in]
                          n623 = Bundle By Name(cluster=T20 {"Frame"=0, "Header Text Color"=0, "Header Background"=8453954, "BodyBackgroundPublic"=16121600, "BodyBackgroundProtected"=16777215, "BodyBackgroundPrivate"=16777215, "Body Text Color"=1, "Frame thickness"=1, "ProtectedPrivateSame"=FALSE, "Icon Header Size"=7, "Font Compression"=enum."Auto", "CapitalOnly"=TRUE} ("Colors"), "Frame"=w1430, "Header Text Color"=w1425, "Header Background"=w1424, "BodyBackgroundPublic"=w1429, "BodyBackgroundProtected"=w1428, "BodyBackgroundPrivate"=w1427, "Body Text Color"=w1425) -> (w1431:T20)
                          n624 = Bundle(cluster=T21 {"Text"="myhedaer", "Allow Only Capital Chars"=TRUE, "Compression"=enum."Auto", "Alignment"=enum."Center"} ("Text"), "Text"=w1426) -> (w1434:T21)  [unwired: 3 out]
                          n625 = Bundle By Name(cluster=T25 {"InterfaceName"="", "InterfaceFolder"=path "", "InterfaceDescription"="", "FolderSuffix"="", "MethodsToCreate"=[], "ParentInterfaces"=[]} ("CreateInterfaceData"), "InterfaceName"=w1408, "InterfaceFolder"=w1402, "InterfaceDescription"=w1401, "ParentInterfaces"=w1399) -> (w1409:T25)
                          n626 = call <resource>:"GDSLvIcon_GenerateIconText.vi"("Text"=w1434, "TextPixelHeight(5-30)"=7, "Foreground color"=w1425, "Background color"=w1424, "error in (no error)"=w1420, "Text Pixel width(32-FrameThicknes*2))"=30) -> ("TextOut"=w1432:u8[][], "error out"=w1417:errorcluster)  [unwired: 2 in, 10 out]
                          n627 = Bundle("Colors"=w1431, "TextOut"=w1432) -> (w1413:cluster{"Colors":T20, "TextOut":u8[][]})  [unwired: 1 out]
                          n628 = call-dynamic "CreateInterface.vi"("ClassWriter.lvclass"=w1437, "ProjectTreePosition(String or Project Item Ref)"=w1411, "CreateInterfaceData"=w1409, "error in (no error)"=w1417, "KeepLvClassRefOpen(False)"=TRUE, "HeaderToApply (take from VIRef or /use 2D-8bit header, Ignored if not wired)"=w1413) -> ("LVClassLibraryRefnum"=w1396:refnum<vi>, "error out"=w1397:errorcluster)  [unwired: 11 in, 1 out]
                          n629 = Bundle By Name(cluster=w1439, "LVClassRef"=w1396) -> (w1440:T15)
                          n630 = call <resource>:"GOOP_ApplyOverlayIconFromClassRef.vi"("error in (no error)"=w1397, "LVClassRef"=w1396) -> ("error out"=w1398:errorcluster)  [unwired: 9 in]
                          n631 = Build Array(w1440) -> (w1438:T15[])
                          n632 = Close Reference(reference=w1396, error in (no error)=w1398) -> (error out=w1395:errorcluster)
                        }
                      }
                    }
                  }
                }
                frame True {
                  n633 = Format Into String(format string="Class %s already exists", w1448) -> (resulting string=w1453:string)  [unwired: 2 in, 1 out]
                  n634 = case shown="False" w1454 {
                    tunnel: w1453 -> [w1465 w1470]
                    tunnel: [w1464 w1470] -> w1441
                    tunnel: w1452 -> [w1462 _]
                    tunnel: w1451 -> [w1461 w1466]
                    tunnel: w1450 -> [w1460 w1469]
                    tunnel: [w1459 w1468] -> w1444
                    tunnel: [w1456 w1467] -> w1445
                    frame False {
                      n635 = invoke class="ProjectItem" method="AddFile"(reference=w1462, error in=w1460, "Path"=w1461) -> (error out=w1459:errorcluster, "AddFile"=w1458:refnum<vi>)  [unwired: 1 in, 2 out]
                      n636 = To More Specific Class(target class=refnum<vi> refnum ("LVClassRef"), reference=w1458) -> (specific class reference=w1456:refnum<vi>)  [unwired: 1 in, 1 out]
                      n637 = Concatenate Strings(w1465, ", but needs to be added into the project" ("string")) -> (w1464:string)
                    }
                    frame True {
                      n638 = call <resource>:"GDSProject_OpenClass.vi"("ClassPath(FilePath/ProjectTreePath/LvCLassRef)"=w1466, "error IO"=w1469) -> ("LVClass.Open"=w1467:refnum<vi>, "error out"=w1468:errorcluster)  [unwired: 16 out]
                    }
                  }
                  n639 = Bundle By Name(cluster=w1447, "LVClassRef"=w1445) -> (w1446:T15)
                  n640 = call <resource>:"GOOP_DebugLogger.vi"("error in (no error)"=w1444, "Data"=w1441, "State"=w1442) -> ("error out"=w1443:errorcluster)  [unwired: 6 in, 2 out]
                  n641 = call <resource>:"UMLEditor createWizardScriptFile_UpdateList.vi"("String"=w1441) -> ()  [unwired: 10 in, 1 out]
                  n642 = Build Array(w1446) -> (w1449:T15[])
                }
              }
              n643 = Greater?(x=w1281, y=1000) -> (0:w1276:bool)
              n644 = Build Array (concatenate)(w1269, w1268) -> (w1267:T15[])
              n645 = Build Array (concatenate)(w1284, w1283) -> (w1282:T15[])
              n646 = Empty Array?(array=w1282) -> (empty?=w1278:bool)
              n647 = Unbundle(w1277) -> ("status"=w1275:bool)  [unwired: 2 out]
              n648 = Compound Arithmetic op=OR(w1278, w1276, w1275) -> (w1279:bool)
            }
            n649 = Bundle By Name(cluster=w1250, "classes"=w1251) -> (w1252:T16)
          }
          frame "UpdateClassPathInDiagramClasses" {
            n650 = Unbundle By Name(w1473) -> ("classes"=w1485:T15[])
            n651 = Unbundle By Name(w1473) -> ("graph"=w1474:refnum<class "Graph.lvclass">)
            n652 = for {
              tunnel: w1485 -> [w1492] mode=indexing
              shift-right: [w1495] -> w1482
              shift-left: w1484 -> [w1497]
              tunnel: w1474 -> [_]
              tunnel: [w1490] -> w1471 mode=indexing
              n653 = Unbundle By Name(w1492) -> ("Class folder"=w1489:path, "Node"=w1488:refnum<class "ClassNode.lvclass">)  [unwired: 1 out]
              n654 = call <vilib>:"Get File Extension.vi"("file"=w1489) -> ("filename without extension"=w1493:string, "lowercase file extension"=w1494:string)  [unwired: 6 in, 3 out]
              n655 = case shown="Default" w1494 {
                tunnel: w1489 -> [_ w1519]
                tunnel: [w1499 w1519] -> w1491
                tunnel: w1493 -> [w1512 _]
                tunnel: w1489 -> [w1513 _]
                frame Default {
                  w1500 = "*.lvclass" ("pattern")
                  n656 = Concatenate Strings(w1512, "*" ("string")) -> (w1510:string)
                  n657 = List Folder(path=w1513, pattern=w1510) -> (path out=w1501:path, folder names=w1509:string[])  [unwired: 2 in, 2 out]
                  n658 = Index Array(array=w1509) -> (element=w1508:string)  [unwired: 1 in]
                  n659 = Build Path(base path=w1501, name or relative path=w1508) -> (appended path=w1507:path)
                  n660 = List Folder(path=w1507, pattern=w1500) -> (path out=w1505:path, filenames=w1506:string[])  [unwired: 2 in, 2 out]
                  n661 = Index Array(array=w1506) -> (element=w1504:string)  [unwired: 1 in]
                  n662 = Build Path(base path=w1505, name or relative path=w1504) -> (appended path=w1503:path)
                  n663 = call <vilib>:"Check if File or Folder Exists.vi"("path"=w1503) -> ("file or folder exists?"=w1502:bool, "dup path"=w1498:path)  [unwired: 8 in, 1 out]
                  n664 = case shown="True" w1502 {
                    tunnel: w1501 -> [w1517 _]
                    tunnel: w1500 -> [w1516 _]
                    tunnel: [w1514 w1518] -> w1499
                    tunnel: w1498 -> [_ w1518]
                    frame False {
                      n665 = call <vilib>:"Recursive File List.vi"("pattern"=w1516, "Folder Path"=w1517) -> ("All Files in Dir"=w1515:path[])  [unwired: 5 in, 4 out]
                      n666 = Index Array(array=w1515) -> (element=w1514:path)  [unwired: 1 in]
                    }
                    frame True {
                    }
                  }
                }
                frame "lvclass" {
                }
              }
              n667 = Bundle By Name(cluster=w1492, "Class folder"=w1491) -> (w1490:T15)
              n668 = call-dynamic "ExternalSetParam.vi"("reference"=w1488, "setParameter"=ExternalSetTypes."ClassPath", "error in (no error)"=w1497, "ClassPath"=w1491) -> ("error out"=w1495:errorcluster)  [unwired: 14 in, 1 out]
            }
            n669 = Unbundle By Name(w1473) -> ("Types"=w1480:refnum<class "ClassNode.lvclass">[])
            n670 = Array Size(array=w1480) -> (size(s)=w1479:i32)
            n671 = case shown="0" w1479 {
              tunnel: ["UpdateAttributesAndMethods" ("y") "CreateTypeDefs" ("y")] -> w1478
              frame 0 {
              }
              frame Default {
              }
            }
            n672 = call <resource>:"UMLEditor setDiagramInfo.vi"("error in (no error)"=w1482, "localVariablesIn"=w1477, "action"=enum16{"Name/Dir", "Unsaved", "Saved"}."Unsaved") -> ("localVariablesOut"=→"localVariables":T3, "error out"=w1476:errorcluster)  [unwired: 2 in, 13 out]
            n673 = call-dynamic "layout.vi"("reference"=w1474, "error in (no error)"=w1476) -> ("error out"=w1475:errorcluster)  [unwired: 16 in, 1 out]
            n674 = Bundle By Name(cluster=w1473, "classes"=w1471) -> (w1472:T16)
          }
          frame "CreateTypeDefs" {
            n675 = Unbundle By Name(w1538) -> ("Types"=w1539:refnum<class "ClassNode.lvclass">[], "graph"=w1521:refnum<class "Graph.lvclass">, "nodes"=w1520:refnum<class "ClassNode.lvclass">[])
            n676 = local read "ClassPath"() -> (w1536:path)
            n677 = for {
              tunnel: w1520 -> [w1563] mode=indexing
              shift-right: [w1558] -> _
              shift-left: w1530 -> [w1562]
              tunnel: [w1556] -> w1529 mode=indexing
              tunnel: [w1554] -> w1527 mode=indexing
              n678 = call <resource>:"ExternalGetParam.vi"("reference"=w1563, "setParameter"=ExternalSetTypes."ClassPath", "error in (no error)"=w1562) -> ("reference out"=w1559:refnum<class "ClassNode.lvclass">, "Path"=w1555:path, "error out"=w1561:errorcluster)  [unwired: 14 out]
              n679 = Strip Path(path=w1555) -> (stripped path=w1554:path)  [unwired: 1 out]
              n680 = call <resource>:"ExternalGetParam.vi"("reference"=w1559, "setParameter"=ExternalSetTypes."Name", "error in (no error)"=w1561) -> ("string"=w1557:string, "error out"=w1558:errorcluster)  [unwired: 15 out]
              n681 = call <resource>:"CommonVIs SterotypeStringParser.vi"("SterotypeStringIn"=w1557) -> ("Name"=w1556:string)  [unwired: 18 out]
            }
            n682 = To Lower Case(string=w1529) -> (all lower case string=w1528:string[])
            n683 = for {
              tunnel: w1539 -> [w1602] mode=indexing
              tunnel: w1536 -> [w1597]
              shift-right: [w1580] -> w1524
              shift-left: w1530 -> [w1595]
              tunnel: w1528 -> [w1591]
              tunnel: w1527 -> [w1583]
              tunnel: [w1579] -> w1526 mode=indexing
              tunnel: [w1578] -> w1525 mode=indexing
              tunnel: [w1577] -> w1522 mode=indexing
              w1572 = ".ctl" ("string")
              n684 = call-dynamic "getClassInfo.vi"("reference"=w1602, "error in (no error)"=w1595) -> ("reference out"=w1601:refnum<class "ClassNode.lvclass">, "className"=w1596:string, "ClassPath"=w1568:path, "error out"=w1600:errorcluster)  [unwired: 8 in, 6 out]
              n685 = Not A Number/Path/Refnum?(number/path/refnum=w1568) -> (NaN/Path/Refnum?=w1575:bool)
              n686 = Empty String/Path?(string/path=w1568) -> (empty?=w1576:bool)
              n687 = call <resource>:"CommonVIs SterotypeStringParser.vi"("SterotypeStringIn"=w1596) -> ("Name"=w1593:string)  [unwired: 18 out]
              n688 = call <resource>:"ExternalGetParam.vi"("reference"=w1601, "setParameter"=ExternalSetTypes."Attributes", "error in (no error)"=w1600) -> ("reference out"=w1598:refnum<class "ClassNode.lvclass">, "error out"=w1594:errorcluster)  [unwired: 15 out]
              n689 = Or(x=w1575, y=w1576) -> (x .or. y?=w1574:bool)
              n690 = call <resource>:"CommonVIs ClassItemStringParser.vi"("ClassItemNameIn"=w1593) -> ("Class"=w1590:string, "Name"=w1578:string)  [unwired: 17 out]
              n691 = Concatenate Strings(w1578, w1572) -> (w1584:string)
              n692 = Build Path(base path=w1597, name or relative path=w1584) -> (appended path=w1587:path)
              n693 = call <vilib>:"Get File Extension.vi"("file"=w1568) -> ("filename without extension"=w1573:string, "dup file"=w1570:path)  [unwired: 6 in, 3 out]
              n694 = To Lower Case(string=w1590) -> (all lower case string=w1589:string)
              n695 = Concatenate Strings(w1573, w1572) -> (w1571:string)
              n696 = Strip Path(path=w1570) -> (stripped path=w1569:path)  [unwired: 1 out]
              n697 = Build Path(base path=w1569, name or relative path=w1571) -> (appended path=w1567:path)
              n698 = Search 1D Array(1D array=w1591, element=w1589) -> (index of element=w1582:i32)  [unwired: 1 out]
              n699 = Index Array(array=w1583, index=w1582) -> (element=w1581:path)
              n700 = Build Path(base path=w1581, name or relative path=w1584) -> (appended path=w1585:path)
              n701 = Greater Or Equal To 0?(x=w1582) -> (x >= 0?=w1588:bool)
              n702 = Select(t=w1585, s=w1588, f=w1587) -> (s? t:f=w1586:path)
              n703 = Select(t=w1586, s=w1574, f=w1567) -> (s? t:f=w1592:path)
              n704 = call-dynamic "ExternalSetParam.vi"("reference"=w1598, "setParameter"=ExternalSetTypes."ClassPath", "error in (no error)"=w1594, "ClassPath"=w1592) -> ("reference out"=w1577:refnum<class "ClassNode.lvclass">, "error out"=w1580:errorcluster)  [unwired: 14 in]
              n705 = File/Directory Info(path=w1592) -> (error out=w1579:errorcluster)  [unwired: 1 in, 6 out]
            }
            n706 = for {
              tunnel: w1526 -> [w1547] mode=indexing
              tunnel: w1525 -> [w1545] mode=indexing
              shift-right: [w1543] -> w1523
              shift-left: w1524 -> [w1544]
              tunnel: w1522 -> [w1542] mode=indexing
              tunnel: w1521 -> [w1541]
              n707 = Format Into String(format string="Creating type: %s", w1545) -> (resulting string=w1540:string)  [unwired: 2 in, 1 out]
              n708 = case shown="Error" w1547 {
                tunnel: w1544 -> [w1548 w1553]
                tunnel: w1542 -> [_ w1552]
                tunnel: w1541 -> [_ w1551]
                tunnel: [w1548 w1550] -> w1543
                frame No Error {
                }
                frame Error {
                  n709 = call <resource>:"UMLEditor SyncCodeFromUml.vi"("Don't Prompt (False)"=TRUE, "error in"=w1553, "graph"=w1551, "selectedNode"=w1552) -> ("error out"=w1550:errorcluster)  [unwired: 7 out]
                }
              }
              n710 = call <resource>:"UMLEditor createWizardScriptFile_UpdateList.vi"("String"=w1540) -> ()  [unwired: 10 in, 1 out]
            }
            n711 = case shown="\"UpdateClassPathInDiagramClasses\"" w1531 {
              tunnel: ["UpdateAttributesAndMethods" ("y") "Done" ("y")] -> w1537
              frame "UpdateClassPathInDiagramClasses" {
              }
              frame Default {
              }
            }
            n712 = local read "localVariables"() -> (w1533:T3)
            n713 = call <resource>:"UMLEditor setDiagramInfo.vi"("error in (no error)"=w1523, "localVariablesIn"=w1533, "action"=enum16{"Name/Dir", "Unsaved", "Saved"}."Unsaved") -> ("localVariablesOut"=w1534:T3, "error out"=w1532:errorcluster)  [unwired: 2 in, 13 out]
            n714 = local write "localVariables"(w1534) -> ()
          }
          frame "UpdateAttributesAndMethods" {
            n715 = Unbundle By Name(w1615) -> ("classes"=w1619:T15[], "Types"=w1613:refnum<class "ClassNode.lvclass">[], "nodes"=w1612:refnum<class "ClassNode.lvclass">[])
            n716 = call <resource>:"CommonVIs_UmlOpenVIRef.vi"() -> ("ProjectNameOut"=w1607:string)  [unwired: 4 in, 7 out]
            n717 = Build Array (concatenate)(w1613, w1612) -> (w1611:refnum<class "ClassNode.lvclass">[])
            n718 = for {
              tunnel: w1611 -> [w1631] mode=indexing
              shift-right: [w1626] -> w1616
              shift-left: w1617 -> [w1630]
              tunnel: [w1625] -> w1604 mode=indexing
              n719 = call <resource>:"ExternalGetParam.vi"("reference"=w1631, "setParameter"=ExternalSetTypes."ClassPath", "error in (no error)"=w1630) -> ("reference out"=w1627:refnum<class "ClassNode.lvclass">, "Path"=w1623:path, "error out"=w1629:errorcluster)  [unwired: 14 out]
              n720 = call <resource>:"ExternalGetParam.vi"("reference"=w1627, "setParameter"=ExternalSetTypes."Name", "error in (no error)"=w1629) -> ("string"=w1624:string, "error out"=w1626:errorcluster)  [unwired: 15 out]
              n721 = call <resource>:"CommonVIs SterotypeStringParser.vi"("SterotypeStringIn"=w1624) -> ("Name"=w1622:string)  [unwired: 18 out]
              n722 = call <resource>:"CommonVIs ClassItemStringParser.vi"("ClassItemNameIn"=w1622) -> ("Name"=w1621:string)  [unwired: 18 out]
              n723 = Bundle(cluster=T31 {"ClassNamn"="", "ClassPath"=path "", "InterfaceClass"=FALSE} ("Cluster"), "ClassNamn"=w1621, "ClassPath"=w1623) -> (w1625:T31)  [unwired: 1 out]
            }
            n724 = call <resource>:"UMLEditor_GetP.vi"("GetProjectRefByName/or Ref"=w1607) -> ("ClassesNamesAndPaths"=w1606:T31[])  [unwired: 1 in, 9 out]
            n725 = call <resource>:"UMLEditor createWizardScriptFile_UpdateList.vi"("String"="Updating classes:" ("format string")) -> ("error out"=w1609:errorcluster)  [unwired: 10 in]
            n726 = Build Array (concatenate)(w1604, w1606) -> (w1605:T31[])
            n727 = for {
              tunnel: w1619 -> [w1655] mode=indexing
              shift-right: [w1652] -> w1618
              shift-left: w1616 -> [w1638]
              tunnel: w1605 -> [w1645]
              tunnel: w1610 -> [w1636]
              tunnel: w1609 -> [_]
              n728 = Unbundle By Name(w1655) -> ("Class folder"=w1642:path, "VirtualMethods"=w1650:bool, "BaseClass"=w1649:bool, "ClassStereotype"=w1644:string, "Node"=w1643:refnum<class "ClassNode.lvclass">, "ClassName"=w1635:string)  [unwired: 1 out]
              n729 = call <resource>:"GOOP_DebugLogger.vi"("error in (no error)"=w1638, "Data"=w1635, "State"=w1636) -> ("error out"=w1637:errorcluster)  [unwired: 6 in, 2 out]
              n730 = call <resource>:"ExternalGetParam.vi"("reference"=w1643, "setParameter"=ExternalSetTypes."Attributes", "error in (no error)"=w1637) -> ("reference out"=w1654:refnum<class "ClassNode.lvclass">, "string"=w1646:string, "error out"=w1653:errorcluster)  [unwired: 14 out]
              n731 = call-dynamic "getClassInfo.vi"("reference"=w1654, "error in (no error)"=w1653) -> ("methods"=w1648:string[], "error out"=w1651:errorcluster)  [unwired: 8 in, 8 out]
              n732 = Concatenate Strings("  Attribute: " ("string"), w1635) -> (w1633:string)
              n733 = Concatenate Strings("  Methods: " ("string"), w1635) -> (w1639:string)
              n734 = call <resource>:"UMLEditor createWizardScriptFile_UpdateList.vi"("String"=w1633) -> ("error out"=w1634:errorcluster)  [unwired: 10 in]
              n735 = stacked-sequence {
                tunnel: [w1668] -> w1652
                tunnel: w1651 -> [w1670]
                tunnel: w1642 -> [w1669]
                tunnel: w1642 -> [w1667]
                tunnel: w1648 -> [w1666]
                tunnel: w1649 -> [w1665]
                tunnel: w1650 -> [w1664]
                tunnel: w1646 -> [w1663]
                tunnel: w1645 -> [w1662]
                tunnel: w1644 -> [w1661]
                tunnel: w1634 -> [_]
                tunnel: w1639 -> [w1656]
                frame #0 {
                  n736 = call <resource>:"ReversedEngineering UpdateAttributes.vi"("ClassPath/LvClassRef"=w1669, "NewAttributes"=w1663, "ClassInfo"=w1662, "error in (no error)"=w1670, "Don't Prompt (False)"=TRUE, "Stereotype"=w1661) -> ("error out"=w1658:errorcluster)  [unwired: 13 out]
                  n737 = call <resource>:"UMLEditor createWizardScriptFile_UpdateList.vi"("error in (no error)"=w1658, "String"=w1656) -> ("error out"=w1657:errorcluster)  [unwired: 9 in]
                  n738 = call <resource>:"ReversedEngineering UpdateClassMethods.vi"("ClassPath/LvClassRef"=w1667, "Methods"=w1666, "error in (no error)"=w1657, "BaseClass"=w1665, "Don'tShowDialog(False)"=TRUE, "UseVirtualMethods(True)"=w1664) -> ("error out"=w1668:errorcluster)  [unwired: 1 in, 12 out]
                }
              }
            }
          }
          frame "FixMethods" {
            n739 = Unbundle By Name(w1677) -> ("classes"=w1676:T15[])
            n740 = for {
              tunnel: w1676 -> [w1690] mode=indexing
              shift-right: [w1681] -> w1674
              shift-left: w1675 -> [w1688]
              tunnel: [w1680] -> w1673
              tunnel: [w1679] -> w1671 mode=indexing
              w1686 = TRUE ("ExcludeDependencies")
              n741 = Unbundle By Name(w1690) -> ("Class folder"=w1689:path)
              n742 = call <resource>:"CommonVIs_UmlOpenVIRef.vi"("error in"=w1688) -> ("error out"=w1692:errorcluster, "AppRefOut"=w1691:refnum<vi>)  [unwired: 3 in, 6 out]
              n743 = call <resource>:"GDSLvClass_OpenClass.vi"("ClassToOpen"=w1689, "error in (no error)"=w1692, "Project/ApplicationRef(If empty, currect active project will be used)"=w1691) -> ("LVClass.Open"=w1687:refnum<vi>, "error out"=w1682:errorcluster)  [unwired: 15 out]
              n744 = invoke class="LVClassLibrary" method="Get All Descendents"(reference=w1687, error in=w1682, "Type"="VI", "Exclude Dependencies"=w1686, "ExcludeBuilds"=w1686, "ExcludeTargets"=w1686) -> (reference out=w1679:refnum<vi>, error out=w1683:errorcluster, "All Descendents"=w1684:refnum<vi>[])  [unwired: 1 in, 4 out]
              n745 = for {
                tunnel: w1684 -> [w1699] mode=indexing
                shift-right: [w1700] -> w1681
                shift-left: w1683 -> [w1698]
                tunnel: [w1693] -> w1680 mode=indexing
                n746 = property class="ProjectItem"(reference=w1699, error in=w1698) -> (error out=w1694:errorcluster, "Reference"=w1697:refnum<vi>)  [unwired: 1 out]
                n747 = property class="VI"(reference=w1697, error in=w1694) -> (reference out=w1693:refnum<vi>, error out=w1695:errorcluster, "VIType"=w1696:T47)
                n748 = case shown="\"Standard VI\"" w1696 {
                  tunnel: [w1701 w1704] -> w1700
                  tunnel: w1693 -> [_ w1703]
                  tunnel: w1695 -> [w1701 w1702]
                  frame Default {
                  }
                  frame "Standard VI" {
                    n749 = call <resource>:"Scripting_FixBrokenVI.vi"("error in (no error)"=w1702, "ViPath/ViName"=w1703) -> ("error out"=w1704:errorcluster)  [unwired: 9 in]
                  }
                }
              }
            }
            n750 = Close Reference(reference=w1673) -> (error out=w1672:errorcluster)  [unwired: 1 in]
            n751 = Close Reference(reference=w1671, error in (no error)=w1672) -> ()  [unwired: 1 out]
          }
          frame "UpdateNodes" {
            n752 = Unbundle By Name(w1705) -> ("graphics"=w1710:refnum<class "Graphics.lvclass">, "grid"=w1711:refnum<class "Grid.lvclass">)
            n753 = Unbundle By Name(w1708) -> ("classes"=w1712:T15[])
            n754 = Unbundle By Name(w1708) -> ("graph"=w1709:refnum<class "Graph.lvclass">)
            n755 = for {
              tunnel: w1712 -> [w1730] mode=indexing
              shift-right: [w1723] -> w1706
              shift-left: w1707 -> [w1715]
              tunnel: w1709 -> [w1722]
              tunnel: w1710 -> [w1721]
              tunnel: w1711 -> [w1720]
              n756 = Unbundle By Name(w1730) -> ("ClassName"=w1719:string, "Class folder"=w1724:path, "Node"=w1714:refnum<class "ClassNode.lvclass">)
              n757 = call <resource>:"ReversedEngineering SyncUmlFromCode.vi"("SyncAction"=ReversedEngineering_SyncUmlFromCodeActions."GetAttributes&MethodsFromCode", "ClassPath"=w1724, "NodeRef"=w1714, "GraphRef"=w1722, "error in (no error)"=w1715, "ClassName(needed for lllbs)"=w1719, "graphics"=w1721, "grid"=w1720) -> ("attributes"=w1717:string, "methods"=w1716:string, "error out"=w1718:errorcluster)  [unwired: 4 in, 5 out]
              n758 = call-dynamic "ExternalSetParam.vi"("reference"=w1714, "setParameter"=ExternalSetTypes."Attributes", "string"=w1717, "error in (no error)"=w1718) -> ("reference out"=w1727:refnum<class "ClassNode.lvclass">, "error out"=w1728:errorcluster)  [unwired: 14 in]
              n759 = call-dynamic "ExternalSetParam.vi"("reference"=w1727, "setParameter"=ExternalSetTypes."Methods", "string"=w1716, "error in (no error)"=w1728) -> ("error out"=w1723:errorcluster)  [unwired: 14 in, 1 out]
            }
          }
          frame "Done" {
            n760 = call <resource>:"UMLEditor createWizardScriptFile_UpdateList.vi"("String"="--- Done ---") -> ()  [unwired: 10 in, 1 out]
          }
        }
        n761 = Unbundle By Name(w57) -> ("status"=w56:bool)
        n762 = Equal?(x=w55, y="Exit") -> (x = y?=w53:bool)
        n763 = Or(x=w53, y=w56) -> (x .or. y?=w52:bool)
      }
    }
    frame Error {
    }
  }
  "error out" <- w4
  n764 = Unbundle By Name(w22) -> ("cancel"=→"Cancelled":bool, "classes"=w5:T15[], "scriptFilePath"=→"pathToScriptFile":path, "My Computer"=w7:refnum<vi>, "ClassWriterRef"=w6:refnum<class "ClassWriter.lvclass">)
  n765 = call <resource>:"ContextHelp_LeavingDialog.vi"("error in (no error)"=w4) -> ()  [unwired: 2 in, 17 out]
  n766 = flat-sequence {
    tunnel: w4 -> [_]
    tunnel: w3 -> [_]
    frame #0 {
      n767 = Wait (ms)(milliseconds to wait=u32 500) -> ()  [unwired: 1 out]
    }
    frame #1 {
      n768 = property on="Tab" class="TabCtl (strict)"("Value"=enum32{"Create", "Config"}."Create" ("Tab")) -> ()  [unwired: 2 in, 2 out]
    }
  }
  n769 = Reverse 1D Array(array=w5) -> (reversed array=w20:T15[])
  n770 = Close Reference(reference=w7) -> ()  [unwired: 1 in, 1 out]
  n771 = call-dynamic "Destroy.vi"("ClassWriter.lvclass"=w6) -> ()  [unwired: 1 in, 18 out]
  n772 = for {
    tunnel: w5 -> [w1740] mode=indexing
    tunnel: [w1738] -> w3
    n773 = Unbundle By Name(w1740) -> ("LVClassRef"=w1739:refnum<vi>)
    n774 = Close Reference(reference=w1739) -> (error out=w1738:errorcluster)  [unwired: 1 in]
  }
  n775 = Index Array(array=w20) -> (element=w19:T15)  [unwired: 1 in]
  n776 = Unbundle By Name(w19) -> ("Class folder"=→"Class folder":path)
